vi "main_locate.vi"() -> ()   [LabVIEW 2023]
uses:
  <vilib>/Math Plots/3D Math Plots/3D Scatter/3D Scatter XCtrl/3D Scatter.xctl
  <vilib>/Math Plots/3D Math Plots/3D Scatter/3D Scatter Datatype/3D Scatter Datatype.lvclass
  subVis/datas.ctl
  subVis/HologramInfo.ctl
  HoloTrackerLib/holoTracker.lvlib
  HoloTrackerLib/CCL_parameters.ctl
  <vilib>/Math Plots/3D Math Plots/3D Scatter/3D Scatter Datatype/Public/Plot Helper (Vector).vi
  subVis/referencesBtns.ctl
  subVis/globState.vi
  <vilib>/Utility/miscctls.llb/LVStringsAndValuesArrayTypeDef_U16.ctl
  <vilib>/Python/Open Venv Python Session.vi
panel:
  out "Status":string
  in  "result tab":enum32{"Holograms", "Localisations", "infos"}(tab)
  out "2D Picture":picture caption="Hologram"
  out "3D Scatter":refnum<class "3D Plot Datatype.lvclass">[](xcontrol)
  out "Threshold":dbl
  out "Std Var":dbl
  out "Mean":dbl
  out "objects positions":sgl[][](array[numeric]) caption="objects positions\nX                           Y                         Z"
  out "t exec (ms)":u32
  in  "Tab Control":enum32{"PATH", "PARAMETERS", "ACTIONS"}(tab)=enum."ACTIONS"
  in  "HoloDir":path=path "C:/TRAVAIL/developpement/imagesHolo/1000im_manip3" caption="Holograms directory"
  in  "PythonVer":string="3.10" caption="Python version"
  in  "Python/Environnement\npath":path
  in  "remove action":enum16{"Subtract", "Division"}(ring)
  in  "Fourier BP filter (pix)":T1={"High pass (0=none)"=15.0, "Low Pass (0=none)"=125.0} {"Low Pass (0=none)" format="%#_6f"}
  in  "CCL parameters":T2={"Threshold ( N x Standard deviation)"=10.0, "Connectivity"=enum."26", "min voxel"=1.0, "max voxel"=0.0} {"max voxel" min=0.0 max=0.0; "min voxel" min=1.0 max=1.0; "Threshold ( N x Standard deviation)" min=1.0 max=100.0}
  in  "Batch threshold":T3(ring)
  in  "Focus":T4={"Type"=enum."SUM_OF_VARIANCE", "Sum size"=15} {"Sum size" min=1 max=100}
  in  "propagation":T5={"distance ini"=0.0, "number of planes"=100, "step"=1e-06} {"step" format="%#_6e"; "distance ini" format="%#_6e"}
  in  "Remove mean Hologram":bool=TRUE
  in  "HoloParam":T6 caption="Holo parameters" {"wavelength" format="%#_6e"}
  in  "hologram to test":u16(ring)
  in  "exitTestMode":bool
  in  "testMode":bool
  in  "CANCEL_BATCH":bool
  in  "EXIT":bool
  in  "BATCH":bool
  in  "Plane number":u16=95 max=200
  in  "Display":T7(ring)
  # "Analyse parameters"
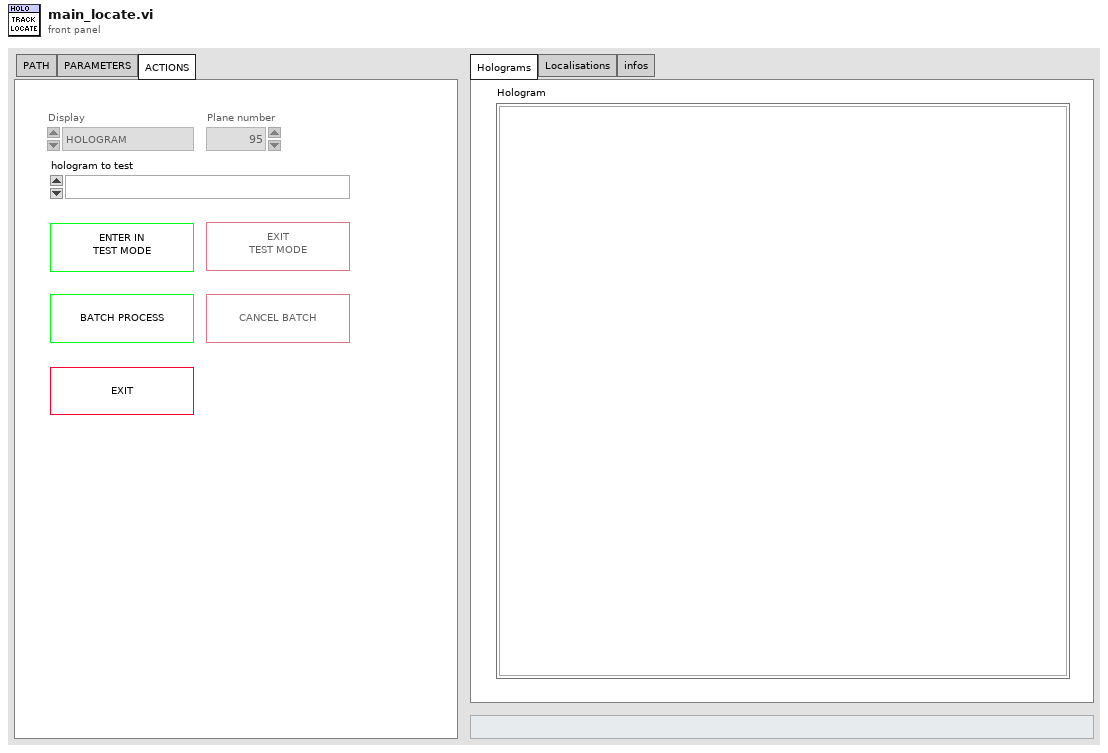
[diagram p1: front panel]
types:
  T1 = cluster{"High pass (0=none)":dbl, "Low Pass (0=none)":dbl}
  T2 = typedef "CCL_parameters.ctl" = cluster{"Threshold ( N x Standard deviation)":dbl, "Connectivity":enum16{"6", "18", "26"}, "min voxel":dbl, "max voxel":dbl}
  T3 = enum16{"compute on 1st hologram", "compute on each hologram"}
  T4 = cluster{"Type":enum16{"SUM_OF_INTENSITY", "SUM_OF_LAPLACIAN", "SUM_OF_VARIANCE", "TENENGRAD"}, "Sum size":i32}
  T5 = cluster{"distance ini":dbl, "number of planes":i32, "step":dbl}
  T6 = typedef "holoTracker.lvlib/HologramInfo.ctl" = cluster{"wavelength":sgl, "optical index":sgl, "Holo size X":i32, "Holo size Y":i32, "pixel size":sgl, "objective magnification":sgl}
  T7 = enum16{"HOLOGRAM", "XY PLANE NUMBER....", "XY MAX PLANE", "XY SUM PLANE", "XZ MAX PLANE", "XZ SUM PLANE", "YZ MAX PLANE", "YZ SUM PLANE"}
  T8 = typedef "referencesBtns.ctl" = cluster{"PythonVer":refnum<vi>, "Python/Environnement\npath":refnum<vi>, "HoloDir":refnum<vi>, "Holo parameters":refnum<vi>, "Remove mean Hologram":refnum<vi>, "propagation":refnum<vi>, "Fourier BP filter (pix)":refnum<vi>, "Focus":refnum<vi>, "Batch thresold ":refnum<vi>, "CCL parameters":refnum<vi>, "testMode":refnum<vi>, "exitTestMode":refnum<vi>, "BATCH":refnum<vi>, "CANCEL_BATCH":refnum<vi>, "EXIT":refnum<vi>, "Plane number":refnum<vi>, "Display":refnum<vi>, "remove action":refnum<vi>}
  T9 = typedef "param_defaut.ctl" = cluster{"PythonVer":string, "Python/Environnement\npath":path, "HoloDir":path, "HoloParam":T6, "Remove mean Hologram":bool, "propagation":cluster{"distance ini":dbl, "number of planes":i32, "step":dbl}, "Fourier BP filter (pix)":cluster{"High pass (0=none)":dbl, "Low Pass (0=none)":dbl}, "Focus":cluster{"Type":enum16{"SUM_OF_INTENSITY", "SUM_OF_LAPLACIAN", "SUM_OF_VARIANCE", "TENENGRAD"}, "Sum size":i32}, "Batch thresold ":enum16{"compute on 1st hologram", "compute on each hologram"}, "CCL parameters":T2}
  T10 = typedef "LVStringsAndValuesArrayTypeDef_U16.ctl" = cluster{"String":string, "Value":u16}[]
  T11 = enum16{"SESSION CLOSED", "WAIT", "TEST WAIT", "TEST IN PROGESS", "BATCH IN PROGRESS"}
  T12 = typedef "datas.ctl" = cluster{"PythonSession":refnum<k35>, "Display":bool, "BinThreshold":sgl, "LIST HOLO BATCH":path[], "Display":sgl[][], "meanHolo":sgl[][], "FEATURES(µm)":sgl[][], "LabelPicture":string, "Status":string, "planeToDisplayFeatures":enum16{"XY", "XZ", "YZ"}, "State":enum16{"SESSION CLOSED", "WAIT", "TEST WAIT", "TEST IN PROGESS", "BATCH IN PROGRESS"}, "HOLO_FILENAME":path, "HOLO_DIRECTORY":path, "LIST HOLO IN DIRECTORY":path[]}
  T13 = cluster{"Remove mean Hologram":bool, "Binarisation thresold ":enum16{"compute on 1st hologram", "compute on each hologram"}, "LIST HOLO BATCH":path[], "HoloDir":path}
  T14 = cluster{"Holo parameters":T6, "propagation":cluster{"distance ini":dbl, "number of planes":i32, "step":dbl}, "Fourier BP filter (pix)":cluster{"High pass (0=none)":dbl, "Low Pass (0=none)":dbl}, "Focus":cluster{"Type":enum16{"SUM_OF_INTENSITY", "SUM_OF_LAPLACIAN", "SUM_OF_VARIANCE", "TENENGRAD"}, "Sum size":i32}, "CCL parameters":T2}
  T15 = cluster{"Display":enum16{"HOLOGRAM", "XY PLANE NUMBER....", "XY MAX PLANE", "XY SUM PLANE", "XZ MAX PLANE", "XZ SUM PLANE", "YZ MAX PLANE", "YZ SUM PLANE"}, "Plane number":u16}
  T16 = cluster{"HOLO_array":sgl[][], "FEATURES(µm)":sgl[][], "Features(pix)":sgl[][], "planeToDisplayFeatures":enum16{"XY", "XZ", "YZ"}, "label":string}
  T17 = cluster{"X":i32, "Y":i32, "Z":i32, "XYsize":i32, "ZSize":i32}
  T18 = typedef "eventvkey.ctl" = enum16{"ASCII", "Enter", "Return", "Shift", "Ctrl", "Alt", "Cmd", "Opt", "Caps", "NumLock", "Clear", "Break", "Up", "Down", "Left", "Right", "Insert", "Delete", "Home", "End", "PageUp", "PageDown", "Escape", "Help", "Pause", "ScrollLock", "F1", "F2", "F3", "F4", "F5", "F6", "F7", "F8", "F9", "F10", "F11", "F12", "F13", "F14", "F15", "F16", "F17", "F18", "F19", "F20", "F21", "F22", "F23", "F24", "Play", "VolumeUp", "VolumeDown", "Mute", "Two Byte Char"}
  T19 = cluster{"Display":enum16{"HOLOGRAM", "XY PLANE NUMBER....", "XY MAX PLANE", "XY SUM PLANE", "XZ MAX PLANE", "XZ SUM PLANE", "YZ MAX PLANE", "YZ SUM PLANE"}, u16}
  T20 = cluster{"PythonVer":string, "Python/Environnement\npath":path, "HoloDir":path, "HoloParam":T6, "Remove mean Hologram":bool, "propagation":cluster{"distance ini":dbl, "number of planes":i32, "step":dbl}, "Fourier BP filter (pix)":cluster{"High pass (0=none)":dbl, "Low Pass (0=none)":dbl}, "Focus":cluster{"Type":enum16{"SUM_OF_INTENSITY", "SUM_OF_LAPLACIAN", "SUM_OF_VARIANCE", "TENENGRAD"}, "Sum size":i32}, "Batch threshold ":enum16{"compute on 1st hologram", "compute on each hologram"}, "CCL parameters":T2}
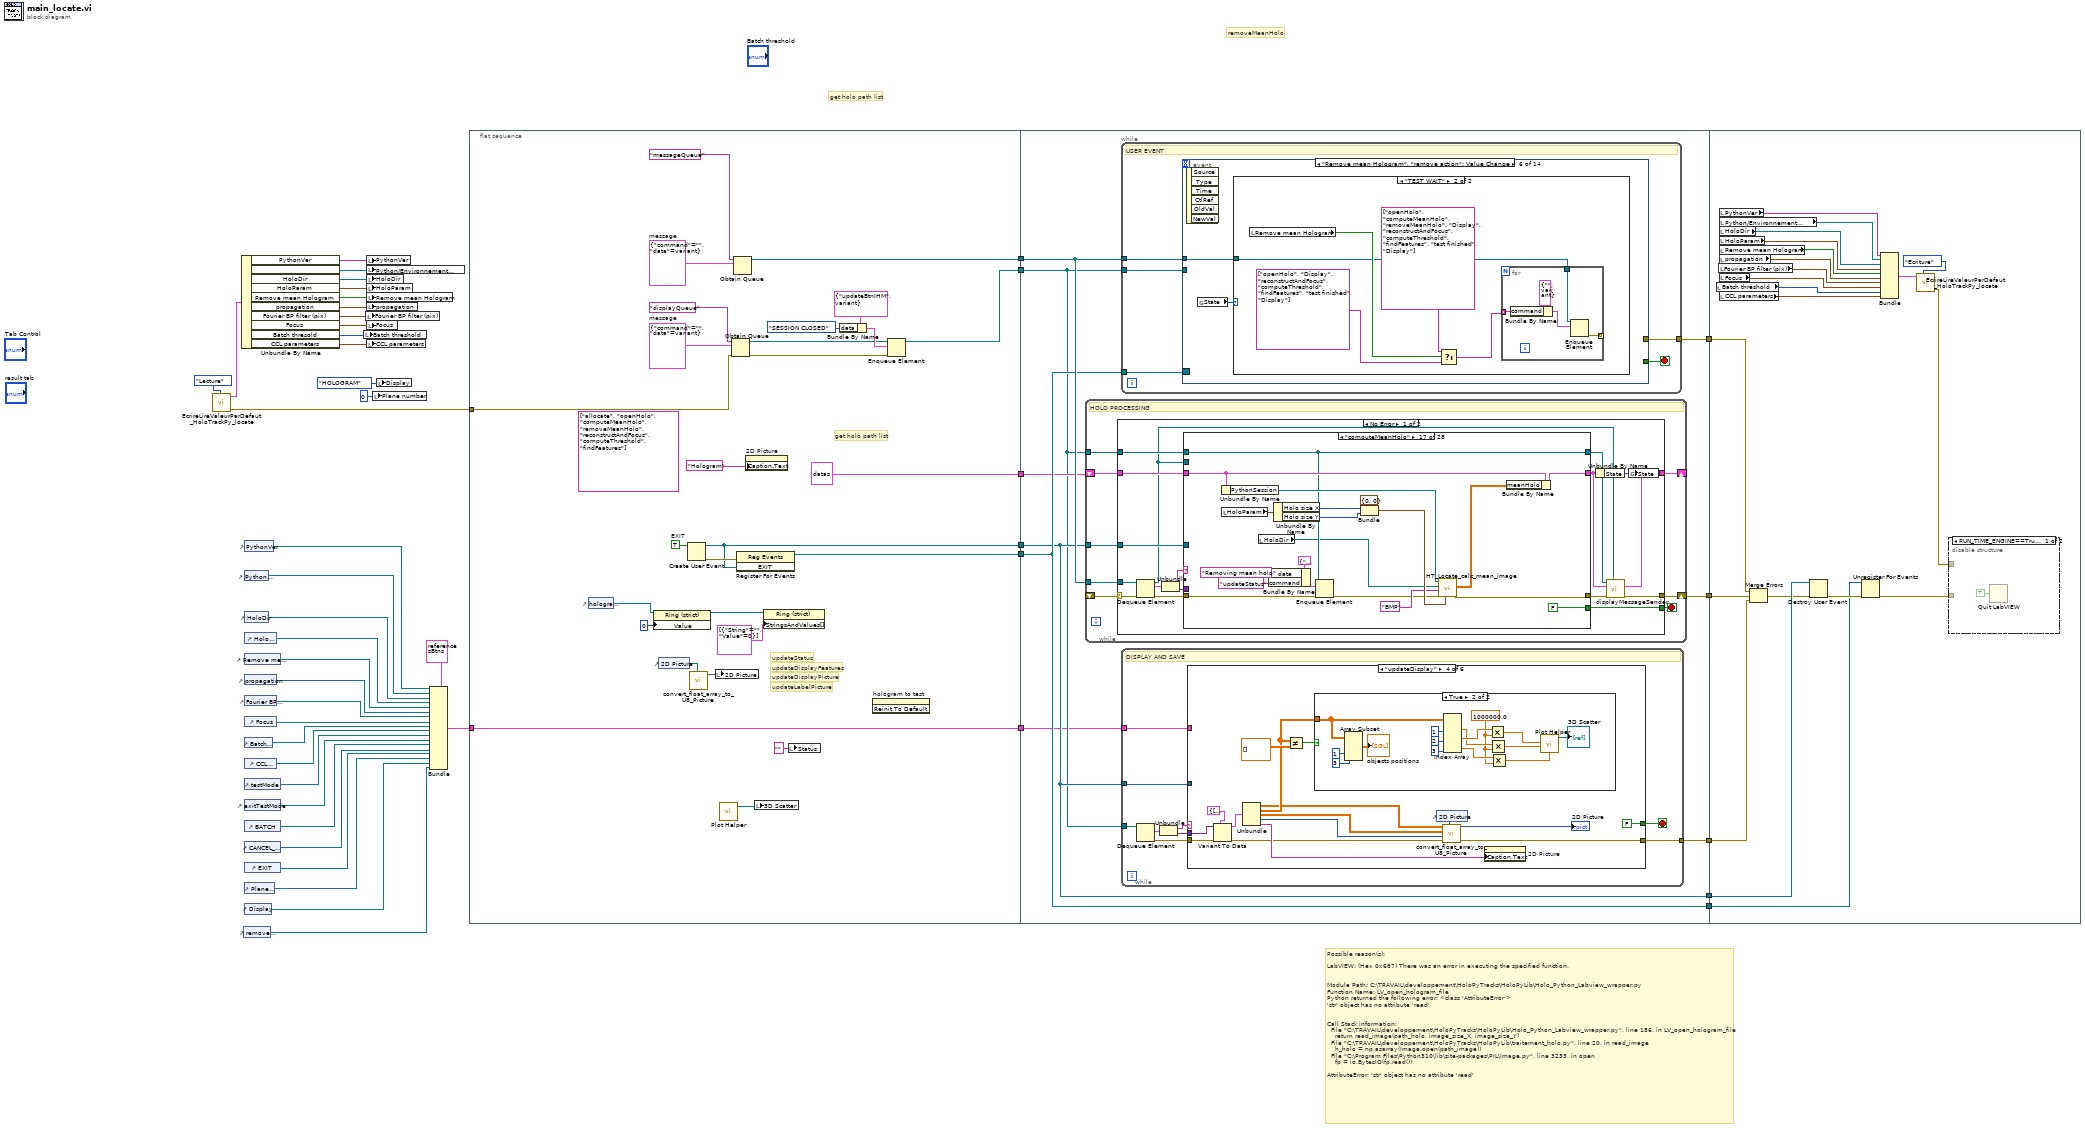
[diagram p0: block diagram]
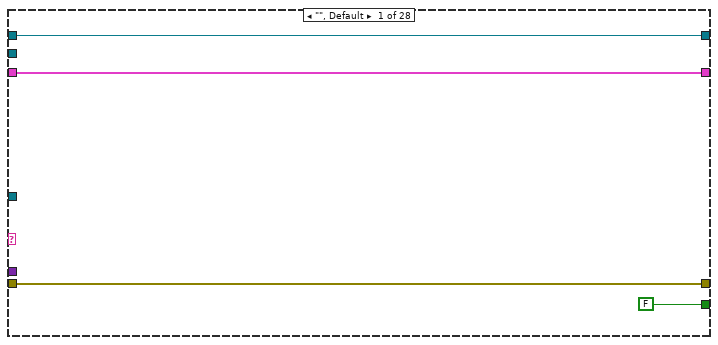
[diagram p2: hidden frame]
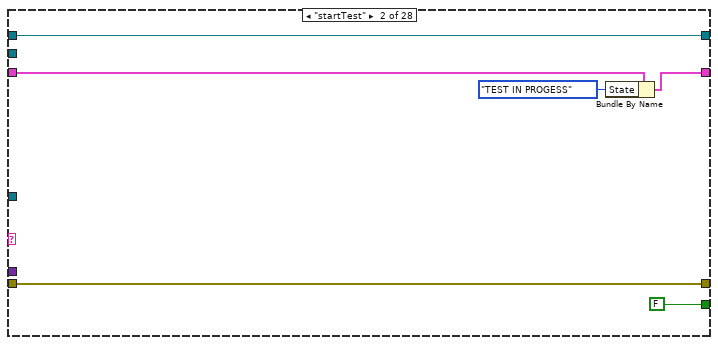
[diagram p3: hidden frame]
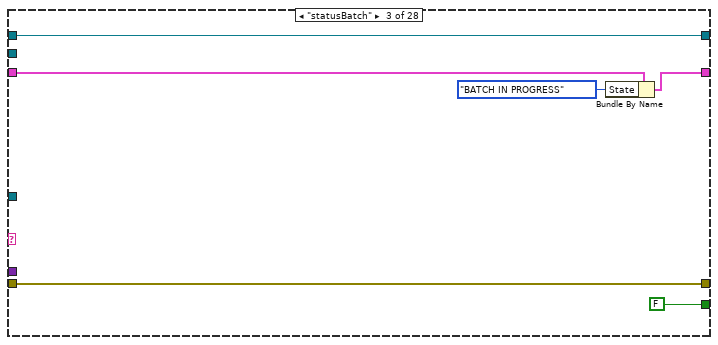
[diagram p4: hidden frame]
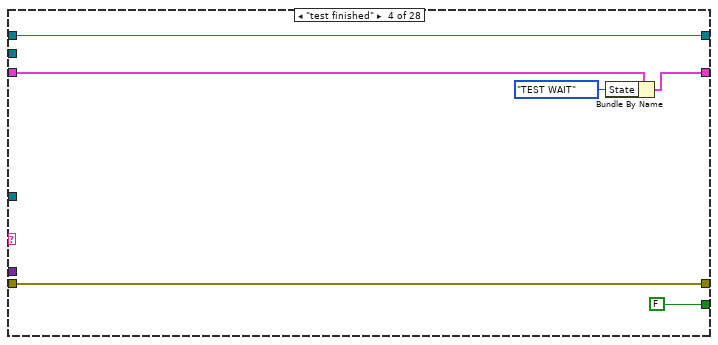
[diagram p5: hidden frame]
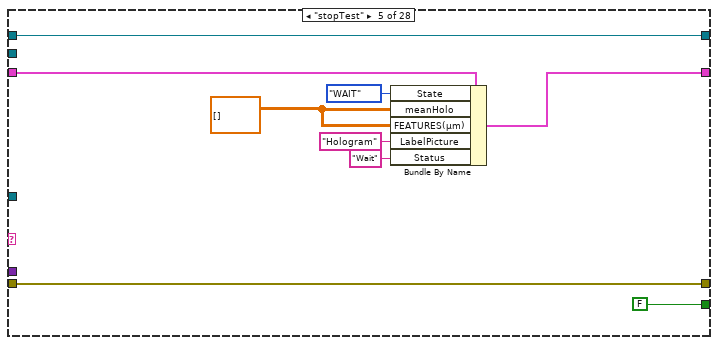
[diagram p6: hidden frame]
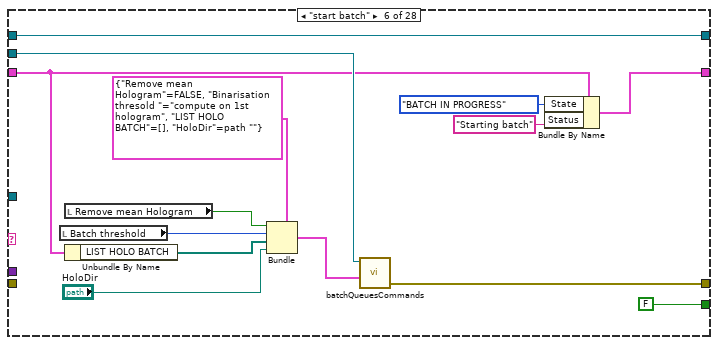
[diagram p7: hidden frame]
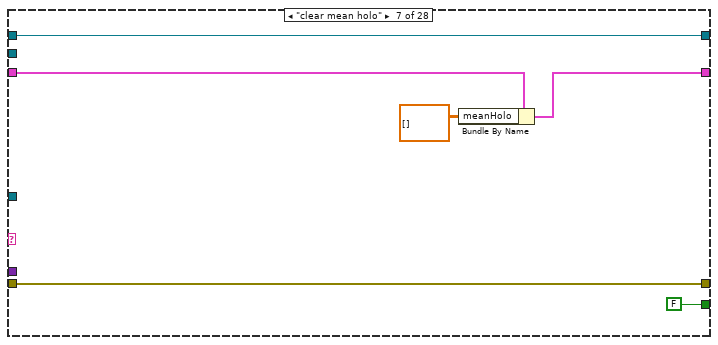
[diagram p8: hidden frame]
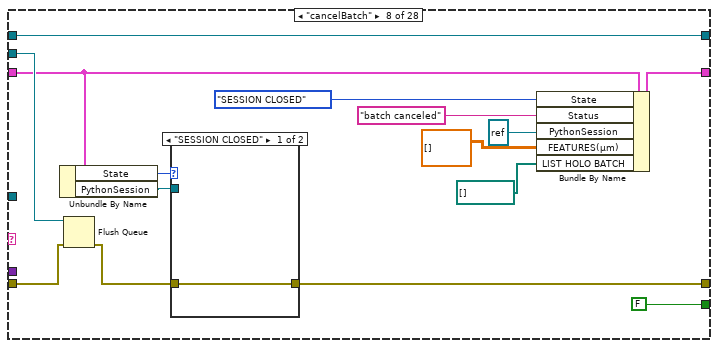
[diagram p9: hidden frame]
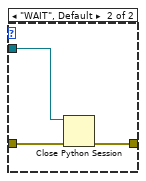
[diagram p10: hidden frame]
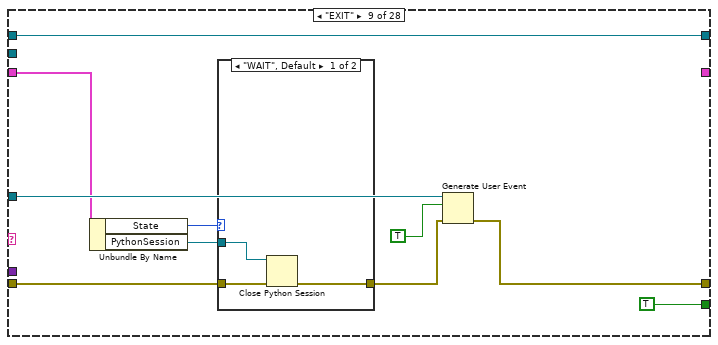
[diagram p11: hidden frame]
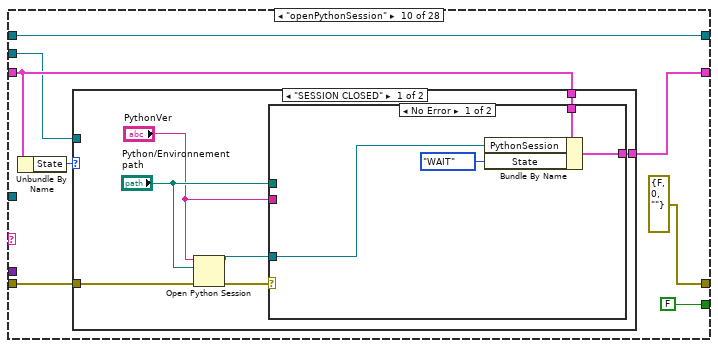
[diagram p13: hidden frame]
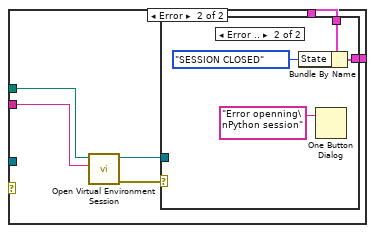
[diagram p14: hidden frame]
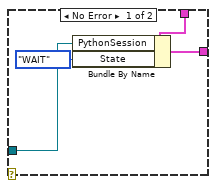
[diagram p15: hidden frame]
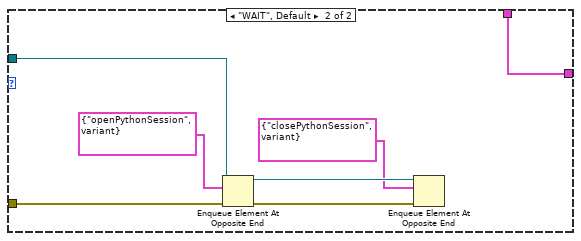
[diagram p16: hidden frame]
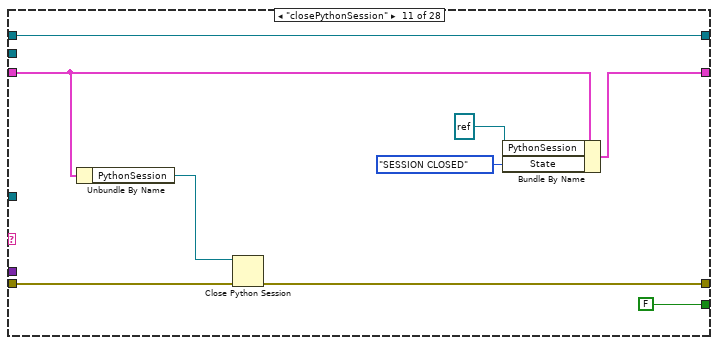
[diagram p17: hidden frame]
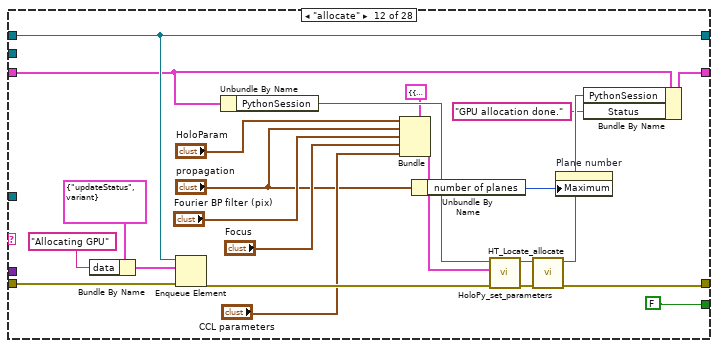
[diagram p18: hidden frame]
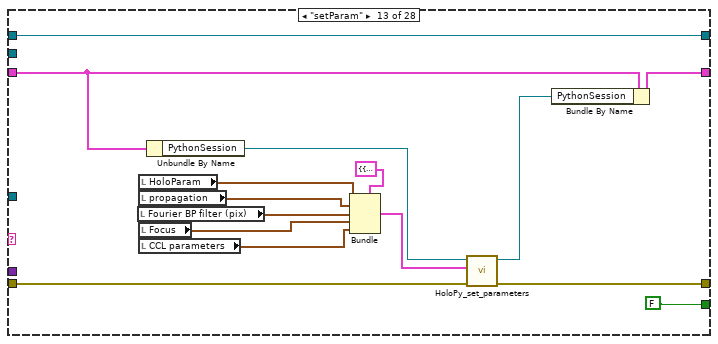
[diagram p19: hidden frame]
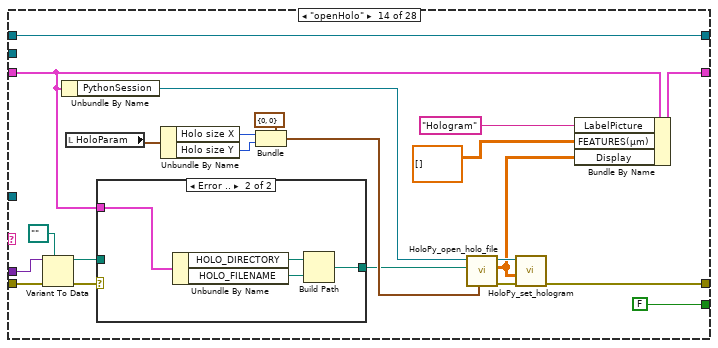
[diagram p20: hidden frame]
diagram:
  # "removeMeanHolo"
  # "get holo path list"
  # "Possible reason(s):\n\nLabVIEW: (Hex 0x687) There was an error in executing the specified function.\n\n\nModule Path: C:\\TRAVAIL\\developpement\\HoloPyTracks\\HoloPyLib\\Holo_Python_Labview_wrapper.py\nFunction Name: LV_open_hologram_file\nPython returned the following error: <class 'AttributeError'>\n'str' object has no attribute 'read'\n\n\nCall Stack information:\n  File \"C:\\TRAVAIL\\developpement\\HoloPyTracks\\HoloPyLib\\Holo_Python_Labview_wrapper.py\", line 186, in LV_open_hologram_file\n    return read_image(path_holo, image_size_X, image_size_Y)\n  File \"C:\\TRAVAIL\\developpement\\HoloPyTracks\\HoloPyLib\\traitement_holo.py\", line 20, in read_image\n    h_holo = np.asarray(Image.open(path_image))\n  File \"C:\\Program Files\\Python310\\lib\\site-packages\\PIL\\Image.py\", line 3233, in open\n    fp = io.BytesIO(fp.read())\n\nAttributeError: 'str' object has no attribute 'read'"
  n1 = call "EcrireLireValeurParDefaut_HoloTrackPy_locate.vi"("Lecture/Ecriture"=enum32{"Lecture", "Ecriture"}."Lecture") -> ("error out"=w34:errorcluster, "ParamOUT"=w36:T9)  [unwired: 7 in, 2 out]
  n2 = Unbundle By Name(w36) -> ("PythonVer"=w31:string, "Python/Environnement\npath"=w30:path, "HoloDir"=w29:path, "HoloParam"=w28:T6, "Remove mean Hologram"=w27:bool, "propagation"=w26:T5, "Fourier BP filter (pix)"=w25:T1, "Focus"=w24:T4, "Batch thresold"=w23:T3, "CCL parameters"=w22:T2)
  n3 = control-ref of="remove action"() -> (w1:refnum<vi>)
  n4 = control-ref of="Plane number"() -> (w3:refnum<vi>)
  n5 = control-ref of="Display"() -> (w2:refnum<vi>)
  n6 = control-ref of="PythonVer"() -> (w32:refnum<vi>)
  n7 = control-ref of="Python/Environnement\npath"() -> (w33:refnum<vi>)
  n8 = control-ref of="HoloDir"() -> (w16:refnum<vi>)
  n9 = control-ref of="Holo parameters"() -> (w15:refnum<vi>)
  n10 = control-ref of="Remove mean Hologram"() -> (w14:refnum<vi>)
  n11 = control-ref of="propagation"() -> (w13:refnum<vi>)
  n12 = control-ref of="Fourier BP filter (pix)"() -> (w12:refnum<vi>)
  n13 = control-ref of="Focus"() -> (w11:refnum<vi>)
  n14 = control-ref of="Batch threshold"() -> (w10:refnum<vi>)
  n15 = control-ref of="CCL parameters"() -> (w9:refnum<vi>)
  n16 = control-ref of="testMode"() -> (w8:refnum<vi>)
  n17 = control-ref of="exitTestMode"() -> (w7:refnum<vi>)
  n18 = control-ref of="BATCH"() -> (w6:refnum<vi>)
  n19 = control-ref of="CANCEL_BATCH"() -> (w5:refnum<vi>)
  n20 = control-ref of="EXIT"() -> (w4:refnum<vi>)
  n21 = local write "Batch threshold"(w23) -> ()
  n22 = local write "Fourier BP filter (pix)"(w25) -> ()
  n23 = local write "PythonVer"(w31) -> ()
  n24 = local write "Python/Environnement\npath"(w30) -> ()
  n25 = local write "HoloDir"(w29) -> ()
  n26 = local write "HoloParam"(w28) -> ()
  n27 = local write "Remove mean Hologram"(w27) -> ()
  n28 = local write "propagation"(w26) -> ()
  n29 = local write "Focus"(w24) -> ()
  n30 = local write "CCL parameters"(w22) -> ()
  n31 = local write "Plane number"(u16 0 ("Plane number")) -> ()
  n32 = local write "Display"(T7."HOLOGRAM" ("Display")) -> ()
  n33 = Bundle(cluster=T8 {"PythonVer"=refnum, "Python/Environnement\npath"=refnum, "HoloDir"=refnum, "Holo parameters"=refnum, "Remove mean Hologram"=refnum, "propagation"=refnum, "Fourier BP filter (pix)"=refnum, "Focus"=refnum, "Batch thresold "=refnum, "CCL parameters"=refnum, "testMode"=refnum, "exitTestMode"=refnum, "BATCH"=refnum, "CANCEL_BATCH"=refnum, "EXIT"=refnum, "Plane number"=refnum, "Display"=refnum, "remove action"=refnum} ("output cluster"), "PythonVer"=w32, "Python/Environnement\npath"=w33, "HoloDir"=w16, "Holo parameters"=w15, "Remove mean Hologram"=w14, "propagation"=w13, "Fourier BP filter (pix)"=w12, "Focus"=w11, "Batch thresold"=w10, "CCL parameters"=w9, "testMode"=w8, "exitTestMode"=w7, "BATCH"=w6, "CANCEL_BATCH"=w5, "EXIT"=w4, "Plane number"=w3, "Display"=w2, "remove action"=w1) -> (w20:T8)
  n34 = flat-sequence {
    tunnel: [w69] -> w46
    tunnel: [w68] -> w45
    tunnel: [w52] -> w44
    tunnel: [T12 {"PythonSession"=refnum, "Display"=FALSE, "BinThreshold"=0.0, "LIST HOLO BATCH"=[], "Display"=[], "meanHolo"=[], "FEATURES(µm)"=[], "LabelPicture"="", "Status"="", "planeToDisplayFeatures"=enum."XY", "State"=enum."SESSION CLOSED", "HOLO_FILENAME"=path "C:/TRAVAIL/developpement/imagesHolo/20um_bon_40X/20um_40x_int_.7ajp1c6t.000000.bmp", "HOLO_DIRECTORY"=path "C:/TRAVAIL/developpement/imagesHolo/20um_bon_40X/20um_40x_int_.7ajp1c6t.000000.bmp", "LIST HOLO IN DIRECTORY"=[]}] -> w43
    tunnel: [w59] -> w37
    tunnel: w20 -> [w59]
    tunnel: w34 -> [w58]
    tunnel: [w51] -> w17
    tunnel: w46 -> [w79]
    tunnel: w45 -> [w81]
    tunnel: w44 -> [w77]
    tunnel: w43 -> [w78]
    tunnel: [w81] -> w42
    tunnel: [w79] -> w41
    tunnel: [w80] -> w40
    tunnel: [w76] -> w39
    tunnel: [w75] -> w38
    tunnel: w37 -> [w74]
    tunnel: w17 -> [w82]
    tunnel: w42 -> [w964]
    tunnel: w41 -> [w963]
    tunnel: w40 -> [w960]
    tunnel: w39 -> [w962]
    tunnel: w38 -> [w961]
    frame #0 {
      (unwired) string[] ["allocate", "openHolo", "computeMeanHolo", "removeMeanHolo", "reconstructAndFocus", "computeThreshold", "findFeatures"]
      w67 = cluster{"command":string, "data":variant} {"command"="", "data"=variant}  # message
      w71 = TRUE  # EXIT
      w72 = cluster{"command":string, "data":variant} {"command"="", "data"=variant}  # message
      # "get holo path list"
      # "updateDisplayFeatures"
      # "updateLabelPicture"
      # "updateDisplayPicture"
      # "updateStatus"
      n35 = control-ref of="hologram to test"() -> (w48:refnum<vi>)
      n36 = property class="Ring (strict)"(reference=w48, "Value"=u16 0) -> (reference out=w47:refnum<vi>)  [unwired: 1 in, 1 out]
      n37 = control-ref of="2D Picture"() -> (w64:refnum<vi>)
      n38 = Create User Event(user event datatype=w71) -> (user event=w69:refnum<user-event>, error out=w70:errorcluster)  [unwired: 1 in]
      n39 = call "convert_float_array_to_U8_Picture.vi"("Pict Refnum"=w64) -> ("new picture"=w63:picture)  [unwired: 9 in, 1 out]
      n40 = local write "2D Picture"(w63) -> ()
      n41 = call-poly <vilib>:"Plot Helper.vi"() -> ("3D Plot lvclass Array out"=w60:refnum<class "3D Plot Datatype.lvclass">[])  [unwired: 6 in, 5 out]
      n42 = Obtain Queue(name (unnamed)="displayQueue", element data type=w67, error in (no error)=w58) -> (queue out=w55:refnum<queue>, error out=w54:errorcluster)  [unwired: 2 in, 1 out]
      n43 = Obtain Queue(name (unnamed)="messageQueue", element data type=w72) -> (queue out=w51:refnum<queue>)  [unwired: 3 in, 2 out]
      n44 = register-events(error in=w70, w69) -> (reference out=w68:refnum<event-registration>)  [unwired: 1 in, 1 out]
      n45 = property on="2D Picture" class="Pict"("Caption.Text"="Hologram" ("Label.Text")) -> ()  [unwired: 2 in, 2 out]
      n46 = local write "3D Scatter"(w60) -> ()
      n47 = property class="Ring (strict)"(reference=w47, "StringsAndValues[]"=T10 [{"String"="", "Value"=0}] ("Strings And Values []")) -> ()  [unwired: 1 in, 2 out]
      n48 = local write "Status"("" ("Status")) -> ()
      n49 = Bundle By Name(cluster=cluster{"command":string, "data":variant} {"command"="updateBtnIHM", "data"=variant} ("element"), "data"=T11."SESSION CLOSED" ("State")) -> (w56:cluster{"command":string, "data":variant})
      n50 = invoke on="hologram to test" class="Ring (strict)" method="Reinit To Default"() -> ()  [unwired: 3 in, 3 out]
      n51 = Enqueue Element(queue=w55, element=w56, error in (no error)=w54) -> (queue out=w52:refnum<queue>)  [unwired: 1 in, 2 out]
    }
    frame #1 {
      n52 = while {
        tunnel: w82 -> [w90]
        tunnel: w79 -> [w88]
        shift-right: [w86] -> _
        shift-left: w78 -> [w87]
        tunnel: w77 -> [w85]
        shift-right: [w84] -> w75
        shift-left: _ -> [w83]
        stop <- w89 stop-if-true
        # "HOLO PROCESSING"
        n53 = case shown="No Error" w83 {
          selector: w83 -> [w98 w699]
          tunnel: w90 -> [w107 w700]
          tunnel: [w102 FALSE] -> w89
          tunnel: w88 -> [w101 _]
          tunnel: w87 -> [w100 w695]
          tunnel: [w94 w695] -> w86
          tunnel: w85 -> [w99 _]
          tunnel: [w96 errorcluster {"status"=FALSE, "code"=0, "source"=""} ("error out")] -> w84
          frame No Error {
            n54 = Dequeue Element(queue=w107, error in (no error)=w98) -> (queue out=w91:refnum<queue>, element=w105:cluster{"command":string, "data":variant}, error out=w106:errorcluster)  [unwired: 1 in, 1 out]
            n55 = Unbundle(w105) -> ("command"=w104:string, "data"=w103:variant)
            n56 = case shown="\"computeMeanHolo\"" w104 {
              tunnel: w106 -> [w109 w113 w119 w125 w131 _ w154 w169 w183 w197 w236 w259 w273 w285 w313 w320 w336 w352 w378 w389 w411 w448 w621 w633 w656 w672 w676 w693]
              tunnel: w103 -> [_ _ _ _ _ _ _ _ _ _ _ _ _ w284 _ _ _ _ _ _ w410 w447 _ w632 w655 w671 _ w692]
              tunnel: [FALSE FALSE FALSE FALSE FALSE FALSE FALSE FALSE TRUE FALSE FALSE FALSE FALSE FALSE FALSE FALSE FALSE FALSE FALSE FALSE FALSE FALSE FALSE FALSE FALSE FALSE FALSE FALSE] -> w102
              tunnel: w101 -> [_ _ _ _ _ _ _ _ w186 _ _ _ _ _ _ _ _ _ _ _ _ _ _ _ _ _ _ _]
              tunnel: w100 -> [w110 w115 w121 w127 w136 w146 w157 w163 w178 w193 w235 w256 w272 w279 w317 w324 w342 w358 w375 w387 w406 w451 w625 w639 w651 w670 w682 w686]
              tunnel: [w110 w114 w120 w126 w135 w148 w156 w172 _ w196 w237 w262 w277 w296 w318 w326 w341 w357 w374 w386 w405 w451 w624 w638 w650 w669 w681 w686] -> w93
              tunnel: w99 -> [w108 w116 w122 w128 w137 w149 w158 w168 w179 w198 w239 w258 w276 w293 w314 w325 w334 w356 w376 w385 w407 w450 w626 w640 w649 w668 w680 w684]
              tunnel: [w109 w113 w119 w125 w131 w150 w154 w161 w180 errorcluster {"status"=FALSE, "code"=0, "source"=""} ("error out") w233 w254 w275 w291 w310 w320 w335 w355 w373 w388 w394 w452 w620 w635 w644 w660 w679 w689] -> w95
              tunnel: w91 -> [_ _ _ _ _ w151 _ w170 _ w192 _ _ _ _ _ _ _ _ _ _ _ _ _ _ _ _ _ _]
              tunnel: [w108 w116 w122 w128 w137 w149 w158 w168 w179 w198 w239 w258 w276 w293 w314 w325 w334 w356 w376 w385 w407 w450 w626 w640 w649 w668 w680 w684] -> w97
              frame "", Default {
              }
              frame "startTest" {
                n57 = Bundle By Name(cluster=w115, "State"=T11."TEST IN PROGESS") -> (w114:T12)
              }
              frame "statusBatch" {
                n58 = Bundle By Name(cluster=w121, "State"=T11."BATCH IN PROGRESS") -> (w120:T12)
              }
              frame "test finished" {
                n59 = Bundle By Name(cluster=w127, "State"=T11."TEST WAIT") -> (w126:T12)
              }
              frame "stopTest" {
                w132 = sgl[][] [] ("meanHolo")
                n60 = Bundle By Name(cluster=w136, "State"=T11."WAIT", "meanHolo"=w132, "FEATURES(µm)"=w132, "LabelPicture"="Hologram", "Status"="Wait") -> (w135:T12)
              }
              frame "start batch" {
                n61 = local read "Batch threshold"() -> (w144:T3)
                n62 = local read "Remove mean Hologram"() -> (w145:bool)
                n63 = Unbundle By Name(w146) -> ("LIST HOLO BATCH"=w143:path[])
                n64 = Bundle(cluster=T13 {"Remove mean Hologram"=FALSE, "Binarisation thresold "=enum."compute on 1st hologram", "LIST HOLO BATCH"=[], "HoloDir"=path ""} ("Batch parameters"), "Remove mean Hologram"=w145, "Binarisation thresold"=w144, "LIST HOLO BATCH"=w143, "HoloDir"="HoloDir") -> (w142:T13)
                n65 = call "batchQueuesCommands.vi"("Batch parameters"=w142, "QueueMessages"=w151) -> ("error out"=w150:errorcluster)  [unwired: 9 in]
                n66 = Bundle By Name(cluster=w146, "State"=T11."BATCH IN PROGRESS", "Status"="Starting batch") -> (w148:T12)
              }
              frame "clear mean holo" {
                n67 = Bundle By Name(cluster=w157, "meanHolo"=sgl[][] []) -> (w156:T12)
              }
              frame "cancelBatch" {
                n68 = Unbundle By Name(w163) -> ("State"=w162:T11, "PythonSession"=w159:refnum<k35>)
                n69 = Flush Queue(queue=w170, error in (no error)=w169) -> (error out=w160:errorcluster)  [unwired: 2 out]
                n70 = case shown="\"SESSION CLOSED\"" w162 {
                  tunnel: [w174 w175] -> w161
                  tunnel: w160 -> [w174 w177]
                  tunnel: w159 -> [_ w176]
                  frame "SESSION CLOSED" {
                  }
                  frame "WAIT", Default {
                    n71 = Close Python Session(session in=w176, error in=w177) -> (11:w175:errorcluster)
                  }
                }
                n72 = Bundle By Name(cluster=w163, "State"=T11."SESSION CLOSED", "Status"="batch canceled" ("command"), "PythonSession"=refnum<k35> refnum, "FEATURES(µm)"=sgl[][] [] ("Holo"), "LIST HOLO BATCH"=path[] []) -> (w172:T12)
              }
              frame "EXIT" {
                n73 = Unbundle By Name(w178) -> ("State"=w184:T11, "PythonSession"=w182:refnum<k35>)
                n74 = case shown="\"WAIT\", Default" w184 {
                  tunnel: w183 -> [w190 w191]
                  tunnel: w182 -> [w189 _]
                  tunnel: [w188 w191] -> w181
                  frame "WAIT", Default {
                    n75 = Close Python Session(session in=w189, error in=w190) -> (11:w188:errorcluster)
                  }
                  frame "SESSION CLOSED" {
                  }
                }
                n76 = Generate User Event(user event=w186, event data cluster=TRUE ("event data"), error in=w181) -> (error out=w180:errorcluster)  [unwired: 1 in, 1 out]
              }
              frame "openPythonSession" {
                n77 = Unbundle By Name(w193) -> ("State"=w194:T11)
                n78 = case shown="\"SESSION CLOSED\"" w194 {
                  tunnel: w197 -> [w206 w231]
                  tunnel: [w203 w225] -> w196
                  tunnel: w193 -> [w200 w225]
                  tunnel: w192 -> [_ w230]
                  frame "SESSION CLOSED" {
                    n79 = Open Python Session(python version="PythonVer", python path="Python/Environnement\npath", 3:w206) -> (session out=w202:refnum<k35>, error out=w205:errorcluster)
                    n80 = case shown="No Error" w205 {
                      tunnel: "Python/Environnement\npath" -> [_ w216]
                      tunnel: "PythonVer" -> [_ w215]
                      tunnel: w200 -> [w210 w213]
                      tunnel: [w209 w212] -> w203
                      tunnel: w202 -> [w208 _]
                      frame No Error {
                        n81 = Bundle By Name(cluster=w210, "PythonSession"=w208, "State"=T11."WAIT") -> (w209:T12)
                      }
                      frame Error {
                        n82 = call-poly <vilib>:"Open Virtual Environment Session.vi"("Python version"=w215, "Env path"=w216) -> ("error out"=w214:errorcluster, "session out"=w211:refnum<k35>)  [unwired: 8 in]
                        n83 = case shown="Error .." w214 {
                          tunnel: w213 -> [w220 w223]
                          tunnel: [w219 w222] -> w212
                          tunnel: w211 -> [w218 _]
                          frame No Error {
                            n84 = Bundle By Name(cluster=w220, "PythonSession"=w218, "State"=T11."WAIT") -> (w219:T12)
                          }
                          frame Error {
                            n85 = Bundle By Name(cluster=w223, "State"=T11."SESSION CLOSED") -> (w222:T12)
                            n86 = One Button Dialog(message="Error openning\nPython session") -> ()  [unwired: 1 in, 1 out]
                          }
                        }
                      }
                    }
                  }
                  frame "WAIT", Default {
                    n87 = Enqueue Element At Opposite End(queue=w230, element=cluster{"command":string, "data":variant} {"command"="openPythonSession", "data"=variant}, error in (no error)=w231) -> (queue out=w227:refnum<queue>, error out=w228:errorcluster)  [unwired: 1 in, 1 out]
                    n88 = Enqueue Element At Opposite End(queue=w227, element=cluster{"command":string, "data":variant} {"command"="closePythonSession", "data"=variant}, error in (no error)=w228) -> ()  [unwired: 1 in, 3 out]
                  }
                }
              }
              frame "closePythonSession" {
                n89 = Unbundle By Name(w235) -> ("PythonSession"=w234:refnum<k35>)
                n90 = Close Python Session(session in=w234, error in=w236) -> (11:w233:errorcluster)
                n91 = Bundle By Name(cluster=w235, "PythonSession"=refnum<k35> refnum, "State"=T11."SESSION CLOSED") -> (w237:T12)
              }
              frame "allocate" {
                n92 = Bundle By Name(cluster=cluster{"command":string, "data":variant} {"command"="updateStatus", "data"=variant} ("element"), "data"="Allocating GPU" ("command")) -> (w257:cluster{"command":string, "data":variant})
                n93 = Enqueue Element(queue=w258, element=w257, error in (no error)=w259) -> (error out=w252:errorcluster)  [unwired: 1 in, 2 out]
                n94 = Unbundle By Name(w256) -> ("PythonSession"=w250:refnum<k35>)
                n95 = Bundle(cluster=T14 {"Holo parameters"={"wavelength"=0.0, "optical index"=0.0, "Holo size X"=0, "Holo size Y"=0, "pixel size"=0.0, "objective magnification"=0.0}, "propagation"={"distance ini"=0.0, "number of planes"=0, "step"=0.0}, "Fourier BP filter (pix)"={"High pass (0=none)"=0.0, "Low Pass (0=none)"=0.0}, "Focus"={"Type"=enum."SUM_OF_INTENSITY", "Sum size"=0}, "CCL parameters"={"Threshold ( N x Standard deviation)"=0.0, "Connectivity"=enum."6", "min voxel"=0.0, "max voxel"=0.0}} ("ParametersIN"), "Holo parameters"="HoloParam", "propagation"="propagation", "Fourier BP filter (pix)"="Fourier BP filter (pix)", "Focus"="Focus", "CCL parameters"="CCL parameters") -> (w248:T14)
                n96 = Unbundle By Name("propagation") -> ("number of planes"=w241:i32)
                n97 = call "HoloPy_set_parameters.vi"("error in (no error)"=w252, "ParametersIN"=w248, "session in"=w250) -> ("error out"=w251:errorcluster, "Refnum out"=w249:refnum<k35>)  [unwired: 6 in, 1 out]
                n98 = call "HT_Locate_allocate.vi"("error in (no error)"=w251, "session in"=w249) -> ("error out"=w254:errorcluster, "Refnum out"=w255:refnum<k35>)  [unwired: 7 in, 1 out]
                n99 = property on="Plane number" class="DigNum (strict)"("Maximum"=w241) -> ()  [unwired: 2 in, 2 out]
                n100 = Bundle By Name(cluster=w256, "PythonSession"=w255, "Status"="GPU allocation done." ("command")) -> (w262:T12)
              }
              frame "setParam" {
                n101 = local read "Fourier BP filter (pix)"() -> (w267:T1)
                n102 = local read "HoloParam"() -> (w269:T6)
                n103 = local read "propagation"() -> (w268:T5)
                n104 = local read "Focus"() -> (w266:T4)
                n105 = local read "CCL parameters"() -> (w265:T2)
                n106 = Unbundle By Name(w272) -> ("PythonSession"=w271:refnum<k35>)
                n107 = Bundle(cluster=T14 {"Holo parameters"={"wavelength"=0.0, "optical index"=0.0, "Holo size X"=0, "Holo size Y"=0, "pixel size"=0.0, "objective magnification"=0.0}, "propagation"={"distance ini"=0.0, "number of planes"=0, "step"=0.0}, "Fourier BP filter (pix)"={"High pass (0=none)"=0.0, "Low Pass (0=none)"=0.0}, "Focus"={"Type"=enum."SUM_OF_INTENSITY", "Sum size"=0}, "CCL parameters"={"Threshold ( N x Standard deviation)"=0.0, "Connectivity"=enum."6", "min voxel"=0.0, "max voxel"=0.0}} ("ParametersIN"), "Holo parameters"=w269, "propagation"=w268, "Fourier BP filter (pix)"=w267, "Focus"=w266, "CCL parameters"=w265) -> (w270:T14)
                n108 = call "HoloPy_set_parameters.vi"("error in (no error)"=w273, "ParametersIN"=w270, "session in"=w271) -> ("error out"=w275:errorcluster, "Refnum out"=w274:refnum<k35>)  [unwired: 6 in, 1 out]
                n109 = Bundle By Name(cluster=w272, "PythonSession"=w274) -> (w277:T12)
              }
              frame "openHolo" {
                n110 = Variant To Data(error in=w285, type=path "" ("appended path"), Variant=w284) -> (data=w280:path, error out=w282:errorcluster)
                n111 = Unbundle By Name(w279) -> ("PythonSession"=w299:refnum<k35>)
                n112 = local read "HoloParam"() -> (w289:T6)
                n113 = case shown="Error .." w282 {
                  tunnel: [w301 w302] -> w281
                  tunnel: w280 -> [w301 _]
                  tunnel: w279 -> [_ w305]
                  frame No Error {
                  }
                  frame Error {
                    n114 = Unbundle By Name(w305) -> ("HOLO_DIRECTORY"=w304:path, "HOLO_FILENAME"=w303:path)
                    n115 = Build Path(base path=w304, name or relative path=w303) -> (appended path=w302:path)
                  }
                }
                n116 = Unbundle By Name(w289) -> ("Holo size X"=w288:i32, "Holo size Y"=w287:i32)
                n117 = Bundle(cluster=cluster{"image_size_X":i32, "image_size_Y":i32} {"image_size_X"=0, "image_size_Y"=0} ("imageSize"), "image_size_X"=w288, "image_size_Y"=w287) -> (w297:cluster{"image_size_X":i32, "image_size_Y":i32})
                n118 = call "HoloPy_open_holo_file.vi"("imageSize"=w297, "image path"=w281, "Refnum in"=w299) -> ("error out"=w295:errorcluster, "Array"=w286:sgl[][], "Refnum out"=w294:refnum<k35>)  [unwired: 6 in]
                n119 = call "HoloPy_set_hologram.vi"("error in (no error)"=w295, "HOLO_array"=w286, "Refnum in"=w294) -> ("error out"=w291:errorcluster)  [unwired: 6 in, 2 out]
                n120 = Bundle By Name(cluster=w279, "LabelPicture"="Hologram" ("Label.Text"), "FEATURES(µm)"=sgl[][] [], "Display"=w286) -> (w296:T12)
              }
              frame "get holo path list" {
                n121 = Unbundle By Name(w317) -> ("PythonSession"=w316:refnum<k35>)
                n122 = local read "HoloDir"() -> (w308:path)
                n123 = call "HoloPy_get_all_image_files_in_directory.vi"("error in (no error)"=w313, "file_extension"="BMP", "holo directory"=w308, "Refnum in"=w316) -> ("error out"=w311:errorcluster, "path"=w306:path[], "Refnum out"=w307:refnum<k35>)  [unwired: 5 in]
                n124 = Index Array(array=w306) -> (element=w309:path)  [unwired: 1 in]
                n125 = control-ref of="hologram to test"() -> (w312:refnum<vi>)
                n126 = call "displayHoloListEnum.vi"("error in (no error)"=w311, "path"=w306, "Ring in"=w312) -> ("error out"=w310:errorcluster)  [unwired: 8 in]
                n127 = Bundle By Name(cluster=w317, "PythonSession"=w307, "LIST HOLO IN DIRECTORY"=w306, "LIST HOLO BATCH"=w306, "HOLO_FILENAME"=w309, "HOLO_DIRECTORY"=w308) -> (w318:T12)
              }
              frame "change holo" {
                n128 = Unbundle By Name(w324) -> ("LIST HOLO IN DIRECTORY"=w323:path[])
                n129 = Index Array(array=w323, index="hologram to test") -> (element=w321:path)
                n130 = Bundle By Name(cluster=w324, "HOLO_FILENAME"=w321) -> (w326:T12)
              }
              frame "computeMeanHolo" {
                n131 = Unbundle By Name(w342) -> ("PythonSession"=w344:refnum<k35>)
                n132 = local read "HoloParam"() -> (w332:T6)
                n133 = local read "HoloDir"() -> (w329:path)
                n134 = Bundle By Name(cluster=cluster{"command":string, "data":variant} {"command"="", "data"=variant} ("element"), "data"="Removing mean holo" ("command"), "command"="updateStatus") -> (w338:cluster{"command":string, "data":variant})
                n135 = Unbundle By Name(w332) -> ("Holo size X"=w331:i32, "Holo size Y"=w330:i32)
                n136 = Enqueue Element(queue=w334, element=w338, error in (no error)=w336) -> (error out=w333:errorcluster)  [unwired: 1 in, 2 out]
                n137 = Bundle(cluster=cluster{"image_size_X":i32, "image_size_Y":i32} {"image_size_X"=0, "image_size_Y"=0} ("imageSize"), "image_size_X"=w331, "image_size_Y"=w330) -> (w345:cluster{"image_size_X":i32, "image_size_Y":i32})
                n138 = call "HT_Locate_calc_mean_image.vi"("imageSize"=w345, "error in (no error)"=w333, "imageFileExtension"="BMP", "directory path"=w329, "Refnum in"=w344) -> ("error out"=w335:errorcluster, "Array"=w328:sgl[][])  [unwired: 4 in, 1 out]
                n139 = Bundle By Name(cluster=w342, "meanHolo"=w328) -> (w341:T12)
              }
              frame "removeMeanHolo" {
                n140 = Unbundle By Name(w358) -> ("PythonSession"=w360:refnum<k35>, "meanHolo"=w359:sgl[][])
                n141 = call "HoloPy_get_hologram.vi"("error in (no error)"=w352, "Refnum in"=w360) -> ("error out"=w362:errorcluster, "HOLO_array"=w348:sgl[][], "Refnum out"=w361:refnum<k35>)  [unwired: 7 in]
                n142 = case shown="\"Division\"" "remove action" {
                  tunnel: w348 -> [w368 w371]
                  tunnel: w359 -> [w367 w370]
                  tunnel: [w364 w369] -> w350
                  frame "Subtract", Default {
                    n143 = Subtract(x=w368, y=w367) -> (x-y=w366:sgl[][])
                    n144 = Array Max & Min(array=w366) -> (min value=w365:sgl)  [unwired: 3 out]
                    n145 = Subtract(x=w366, y=w365) -> (x-y=w364:sgl[][])
                  }
                  frame "Division" {
                    n146 = Divide(x=w371, y=w370) -> (x/y=w369:sgl[][])
                  }
                }
                n147 = call "HoloPy_set_hologram.vi"("error in (no error)"=w362, "HOLO_array"=w350, "Refnum in"=w361) -> ("error out"=w355:errorcluster, "Refnum out"=w351:refnum<k35>)  [unwired: 6 in, 1 out]
                n148 = Bundle By Name(cluster=w358, "PythonSession"=w351, "LabelPicture"="Hologram", "planeToDisplayFeatures"=enum16{"XY", "XZ", "YZ"}."XY", "Display"=w350) -> (w357:T12)
              }
              frame "reconstructAndFocus" {
                n149 = Unbundle By Name(w375) -> ("PythonSession"=w377:refnum<k35>)
                n150 = call "HoloPy_volume_and_focus.vi"("error in (no error)"=w378, "Refnum in"=w377) -> ("error out"=w373:errorcluster, "Refnum out"=w372:refnum<k35>)  [unwired: 7 in, 1 out]
                n151 = Bundle By Name(cluster=w375, "PythonSession"=w372) -> (w374:T12)
              }
              frame "computeThreshold" {
                n152 = local read "CCL parameters"() -> (w384:T2)
                n153 = Unbundle By Name(w387) -> ("PythonSession"=w392:refnum<k35>)
                n154 = Unbundle By Name(w384) -> ("Threshold ( N x Standard deviation)"=w383:dbl)
                n155 = call "HoloPy_get_mean_std_var_volume.vi"("error in (no error)"=w389, "Refnum in"=w392) -> ("error out"=w388:errorcluster, "data volume"=w391:cluster{"mean":dbl, "std var":dbl})  [unwired: 7 in, 1 out]
                n156 = Unbundle By Name(w391) -> ("mean"=w380:dbl, "std var"=w382:dbl)
                "Std Var" <- w382
                "Mean" <- w380
                n157 = Multiply(x=w383, y=w382) -> (x*y=w390:dbl)
                n158 = Add(x=w380, y=w390) -> (x+y=w381:dbl)
                "Threshold" <- w381
                n159 = Bundle By Name(cluster=w387, "BinThreshold"=w381) -> (w386:T12)
              }
              frame "findFeatures" {
                n160 = Unbundle By Name(w406) -> ("LIST HOLO BATCH"=w403:path[], "PythonSession"=w408:refnum<k35>, "BinThreshold"=w409:sgl)
                n161 = Variant To Data(error in=w411, type=cluster{"imageNumber":u32, "Display":bool} {"imageNumber"=0, "Display"=TRUE}, Variant=w410) -> (data=w398:cluster{"imageNumber":u32, "Display":bool}, error out=w399:errorcluster)
                n162 = case shown="Error .." w399 {
                  tunnel: w398 -> [w418 _]
                  tunnel: [w417 u32 0 ("imageNumber")] -> w397
                  tunnel: [w416 TRUE ("Display")] -> w396
                  frame No Error {
                    n163 = Unbundle(w418) -> ("imageNumber"=w417:u32, "Display"=w416:bool)
                  }
                  frame Error {
                  }
                }
                n164 = Array Size(array=w403) -> (size(s)=w400:i32)
                n165 = Equal To 0?(x=w397) -> (x = 0?=w402:bool)
                n166 = call "HoloPy_Find_Features.vi"("imageNumber"=w397, "Threshold"=w409, "Refnum in"=w408) -> ("error out"=w394:errorcluster, "FEATURES(µm)"=w395:sgl[][])  [unwired: 6 in, 1 out]
                n167 = case shown="True" w402 {
                  tunnel: w395 -> [w426 w439]
                  tunnel: [w421 w427] -> w401
                  tunnel: w397 -> [_ w435]
                  tunnel: w400 -> [_ w436]
                  frame True {
                    n168 = Array Size(array=w426) -> (size(s)=w425:i32[])
                    n169 = Index Array(array=w425) -> (element=w424:i32)  [unwired: 1 in]
                    n170 = Number To Decimal String(number=w424) -> (decimal integer string=w422:string)  [unwired: 1 in]
                    n171 = Concatenate Strings(w422, " features found.") -> (w421:string)
                  }
                  frame False {
                    n172 = Array Size(array=w439) -> (size(s)=w438:i32[])
                    n173 = Number To Decimal String(number=w436) -> (decimal integer string=w431:string)  [unwired: 1 in]
                    n174 = Number To Decimal String(number=w435) -> (decimal integer string=w433:string)  [unwired: 1 in]
                    n175 = Index Array(array=w438) -> (element=w437:i32)  [unwired: 1 in]
                    n176 = Number To Decimal String(number=w437) -> (decimal integer string=w429:string)  [unwired: 1 in]
                    n177 = Concatenate Strings("Holo n°", w433, "/", w431, ". " ("string"), w429, " features found.") -> (w427:string)
                  }
                }
                n178 = flat-sequence {
                  tunnel: w394 -> [_]
                  frame #0 {
                    n179 = Tick Count (ms)() -> (millisecond timer value=w414:u32)
                    n180 = feedback #1() -> (w415:u32)  [unwired: 1 in]
                    n181 = feedback-in #1(w414) -> ()
                    n182 = Subtract(x=w414, y=w415) -> (x-y=→"t exec (ms)":u32)
                  }
                }
                n183 = Bundle By Name(cluster=w406, "FEATURES(µm)"=w395, "Display"=w396, "Status"=w401) -> (w405:T12)
              }
              frame "Display" {
                n184 = Unbundle By Name(w451) -> ("PythonSession"=w453:refnum<k35>, "FEATURES(µm)"=w449:sgl[][])
                n185 = local read "Display"() -> (w440:T7)
                n186 = Variant To Data(error in=w448, type=T15 {"Display"=enum."HOLOGRAM", "Plane number"=0} ("output cluster"), Variant=w447) -> (data=w445:T15, error out=w443:errorcluster)
                n187 = Unbundle(w445) -> ("Display"=w442:T7, "Plane number"=w444:u16)
                n188 = Select(t=w440, s=w443, f=w442) -> (s? t:f=w441:T7)
                n189 = case shown="\"HOLOGRAM\", Default" w441 {
                  tunnel: w453 -> [w474 w481 w501 w520 w540 w560 w580 w600]
                  tunnel: [w473 w497 w517 w537 w557 w577 w597 w617] -> w452
                  tunnel: w450 -> [w472 w496 w516 w536 w556 w576 w596 w616]
                  tunnel: w449 -> [w459 w485 w505 w525 w545 w565 w585 w605]
                  tunnel: w444 -> [_ w475 _ _ _ _ _ _]
                  frame "HOLOGRAM", Default {
                    n190 = call "HoloPy_get_hologram.vi"("Refnum in"=w474) -> ("error out"=w467:errorcluster, "HOLO_array"=w463:sgl[][])  [unwired: 8 in, 1 out]
                    n191 = local read "propagation"() -> (w471:T5)
                    n192 = local read "HoloParam"() -> (w468:T6)
                    n193 = Unbundle By Name(w468) -> ("pixel size"=w470:sgl, "objective magnification"=w469:sgl)
                    n194 = Unbundle By Name(w471) -> ("step"=w458:dbl)
                    n195 = Divide(x=w470, y=w469) -> (x/y=w457:sgl)
                    n196 = call "scaleFeaturesPositions_um_pix.vi"("error in (no error)"=w467, "dXY"=w457, "dZ"=w458, "FEATURES(µm)"=w459) -> ("error out"=w466:errorcluster, "Features(pix)"=w462:sgl[][])  [unwired: 6 in]
                    n197 = Bundle(cluster=T16 {"HOLO_array"=[], "FEATURES(µm)"=[], "Features(pix)"=[], "planeToDisplayFeatures"=enum."XY", "label"=""} ("output cluster"), "HOLO_array"=w463, "FEATURES(µm)"=w459, "Features(pix)"=w462, "planeToDisplayFeatures"=enum16{"XY", "XZ", "YZ"}."XY", "label"="Hologram" ("command")) -> (w461:T16)
                    n198 = Bundle By Name(cluster=cluster{"command":string, "data":variant} {"command"="updateDisplay", "data"=variant} ("element"), "data"=w461) -> (w464:cluster{"command":string, "data":variant})
                    n199 = Enqueue Element(queue=w472, element=w464, error in (no error)=w466) -> (error out=w473:errorcluster)  [unwired: 1 in, 2 out]
                  }
                  frame "XY PLANE NUMBER...." {
                    n200 = call "HoloPy_get_reconstruction_plane.vi"("plane number"=w475, "Refnum in"=w481) -> ("error out"=w480:errorcluster, "HOLO_array"=w479:sgl[][])  [unwired: 7 in, 1 out]
                    n201 = local read "propagation"() -> (w495:T5)
                    n202 = local read "HoloParam"() -> (w492:T6)
                    n203 = Unbundle By Name(w492) -> ("pixel size"=w494:sgl, "objective magnification"=w493:sgl)
                    n204 = Number To Decimal String(number=w475) -> (decimal integer string=w478:string)  [unwired: 1 in]
                    n205 = Unbundle By Name(w495) -> ("step"=w484:dbl)
                    n206 = Concatenate Strings("Hologram plane number " ("Label.Text"), w478) -> (w476:string)
                    n207 = Divide(x=w494, y=w493) -> (x/y=w483:sgl)
                    n208 = call "scaleFeaturesPositions_um_pix.vi"("error in (no error)"=w480, "dXY"=w483, "dZ"=w484, "FEATURES(µm)"=w485) -> ("error out"=w491:errorcluster, "Features(pix)"=w488:sgl[][])  [unwired: 6 in]
                    n209 = Bundle(cluster=T16 {"HOLO_array"=[], "FEATURES(µm)"=[], "Features(pix)"=[], "planeToDisplayFeatures"=enum."XY", "label"=""} ("output cluster"), "HOLO_array"=w479, "FEATURES(µm)"=w485, "Features(pix)"=w488, "planeToDisplayFeatures"=enum16{"XY", "XZ", "YZ"}."XY", "label"=w476) -> (w487:T16)
                    n210 = Bundle By Name(cluster=cluster{"command":string, "data":variant} {"command"="updateDisplay", "data"=variant} ("element"), "data"=w487) -> (w489:cluster{"command":string, "data":variant})
                    n211 = Enqueue Element(queue=w496, element=w489, error in (no error)=w491) -> (error out=w497:errorcluster)  [unwired: 1 in, 2 out]
                  }
                  frame "XY MAX PLANE" {
                    n212 = call "HoloPy_max_XY_planes_from_volume.vi"("Refnum in"=w501) -> ("error out"=w499:errorcluster, "XY Plane"=w500:sgl[][])  [unwired: 8 in, 1 out]
                    n213 = local read "propagation"() -> (w515:T5)
                    n214 = local read "HoloParam"() -> (w512:T6)
                    n215 = Unbundle By Name(w512) -> ("pixel size"=w514:sgl, "objective magnification"=w513:sgl)
                    n216 = Unbundle By Name(w515) -> ("step"=w504:dbl)
                    n217 = Divide(x=w514, y=w513) -> (x/y=w503:sgl)
                    n218 = call "scaleFeaturesPositions_um_pix.vi"("error in (no error)"=w499, "dXY"=w503, "dZ"=w504, "FEATURES(µm)"=w505) -> ("error out"=w511:errorcluster, "Features(pix)"=w508:sgl[][])  [unwired: 6 in]
                    n219 = Bundle(cluster=T16 {"HOLO_array"=[], "FEATURES(µm)"=[], "Features(pix)"=[], "planeToDisplayFeatures"=enum."XY", "label"=""} ("output cluster"), "HOLO_array"=w500, "FEATURES(µm)"=w505, "Features(pix)"=w508, "planeToDisplayFeatures"=enum16{"XY", "XZ", "YZ"}."XY", "label"="XY max focus plane projection" ("Label.Text")) -> (w507:T16)
                    n220 = Bundle By Name(cluster=cluster{"command":string, "data":variant} {"command"="updateDisplay", "data"=variant} ("element"), "data"=w507) -> (w509:cluster{"command":string, "data":variant})
                    n221 = Enqueue Element(queue=w516, element=w509, error in (no error)=w511) -> (error out=w517:errorcluster)  [unwired: 1 in, 2 out]
                  }
                  frame "XY SUM PLANE" {
                    n222 = call "HoloPy_sum_XY_planes_from_volume.vi"("Refnum in"=w520) -> ("error out"=w518:errorcluster, "XY Plane"=w519:sgl[][])  [unwired: 8 in, 1 out]
                    n223 = local read "propagation"() -> (w535:T5)
                    n224 = local read "HoloParam"() -> (w532:T6)
                    n225 = Unbundle By Name(w532) -> ("pixel size"=w534:sgl, "objective magnification"=w533:sgl)
                    n226 = Unbundle By Name(w535) -> ("step"=w524:dbl)
                    n227 = Divide(x=w534, y=w533) -> (x/y=w523:sgl)
                    n228 = call "scaleFeaturesPositions_um_pix.vi"("error in (no error)"=w518, "dXY"=w523, "dZ"=w524, "FEATURES(µm)"=w525) -> ("error out"=w531:errorcluster, "Features(pix)"=w528:sgl[][])  [unwired: 6 in]
                    n229 = Bundle(cluster=T16 {"HOLO_array"=[], "FEATURES(µm)"=[], "Features(pix)"=[], "planeToDisplayFeatures"=enum."XY", "label"=""} ("output cluster"), "HOLO_array"=w519, "FEATURES(µm)"=w525, "Features(pix)"=w528, "planeToDisplayFeatures"=enum16{"XY", "XZ", "YZ"}."XY", "label"="XY sum focus plane projection" ("Label.Text")) -> (w527:T16)
                    n230 = Bundle By Name(cluster=cluster{"command":string, "data":variant} {"command"="updateDisplay", "data"=variant} ("element"), "data"=w527) -> (w529:cluster{"command":string, "data":variant})
                    n231 = Enqueue Element(queue=w536, element=w529, error in (no error)=w531) -> (error out=w537:errorcluster)  [unwired: 1 in, 2 out]
                  }
                  frame "XZ MAX PLANE" {
                    n232 = call "HoloPy_max_XZ_planes_from_volume.vi"("Refnum in"=w540) -> ("error out"=w538:errorcluster, "XZ Plane"=w539:sgl[][])  [unwired: 8 in, 1 out]
                    n233 = local read "propagation"() -> (w555:T5)
                    n234 = local read "HoloParam"() -> (w552:T6)
                    n235 = Unbundle By Name(w552) -> ("pixel size"=w554:sgl, "objective magnification"=w553:sgl)
                    n236 = Unbundle By Name(w555) -> ("step"=w544:dbl)
                    n237 = Divide(x=w554, y=w553) -> (x/y=w543:sgl)
                    n238 = call "scaleFeaturesPositions_um_pix.vi"("error in (no error)"=w538, "dXY"=w543, "dZ"=w544, "FEATURES(µm)"=w545) -> ("error out"=w551:errorcluster, "Features(pix)"=w548:sgl[][])  [unwired: 6 in]
                    n239 = Bundle(cluster=T16 {"HOLO_array"=[], "FEATURES(µm)"=[], "Features(pix)"=[], "planeToDisplayFeatures"=enum."XY", "label"=""} ("output cluster"), "HOLO_array"=w539, "FEATURES(µm)"=w545, "Features(pix)"=w548, "planeToDisplayFeatures"=enum16{"XY", "XZ", "YZ"}."XZ", "label"="XZ  max focus plane projection" ("Label.Text")) -> (w547:T16)
                    n240 = Bundle By Name(cluster=cluster{"command":string, "data":variant} {"command"="updateDisplay", "data"=variant} ("element"), "data"=w547) -> (w549:cluster{"command":string, "data":variant})
                    n241 = Enqueue Element(queue=w556, element=w549, error in (no error)=w551) -> (error out=w557:errorcluster)  [unwired: 1 in, 2 out]
                  }
                  frame "XZ SUM PLANE" {
                    n242 = call "HoloPy_sum_XZ_planes_from_volume.vi"("Refnum in"=w560) -> ("error out"=w558:errorcluster, "XZ Plane"=w559:sgl[][])  [unwired: 8 in, 1 out]
                    n243 = local read "propagation"() -> (w575:T5)
                    n244 = local read "HoloParam"() -> (w572:T6)
                    n245 = Unbundle By Name(w572) -> ("pixel size"=w574:sgl, "objective magnification"=w573:sgl)
                    n246 = Unbundle By Name(w575) -> ("step"=w564:dbl)
                    n247 = Divide(x=w574, y=w573) -> (x/y=w563:sgl)
                    n248 = call "scaleFeaturesPositions_um_pix.vi"("error in (no error)"=w558, "dXY"=w563, "dZ"=w564, "FEATURES(µm)"=w565) -> ("error out"=w571:errorcluster, "Features(pix)"=w568:sgl[][])  [unwired: 6 in]
                    n249 = Bundle(cluster=T16 {"HOLO_array"=[], "FEATURES(µm)"=[], "Features(pix)"=[], "planeToDisplayFeatures"=enum."XY", "label"=""} ("output cluster"), "HOLO_array"=w559, "FEATURES(µm)"=w565, "Features(pix)"=w568, "planeToDisplayFeatures"=enum16{"XY", "XZ", "YZ"}."XZ", "label"="XZ  sum focus plane projection" ("Label.Text")) -> (w567:T16)
                    n250 = Bundle By Name(cluster=cluster{"command":string, "data":variant} {"command"="updateDisplay", "data"=variant} ("element"), "data"=w567) -> (w569:cluster{"command":string, "data":variant})
                    n251 = Enqueue Element(queue=w576, element=w569, error in (no error)=w571) -> (error out=w577:errorcluster)  [unwired: 1 in, 2 out]
                  }
                  frame "YZ MAX PLANE" {
                    n252 = call "HoloPy_max_YZ_planes_from_volume.vi"("Refnum in"=w580) -> ("error out"=w578:errorcluster, "YZ Plane"=w579:sgl[][])  [unwired: 8 in, 1 out]
                    n253 = local read "propagation"() -> (w595:T5)
                    n254 = local read "HoloParam"() -> (w592:T6)
                    n255 = Unbundle By Name(w592) -> ("pixel size"=w594:sgl, "objective magnification"=w593:sgl)
                    n256 = Unbundle By Name(w595) -> ("step"=w584:dbl)
                    n257 = Divide(x=w594, y=w593) -> (x/y=w583:sgl)
                    n258 = call "scaleFeaturesPositions_um_pix.vi"("error in (no error)"=w578, "dXY"=w583, "dZ"=w584, "FEATURES(µm)"=w585) -> ("error out"=w591:errorcluster, "Features(pix)"=w588:sgl[][])  [unwired: 6 in]
                    n259 = Bundle(cluster=T16 {"HOLO_array"=[], "FEATURES(µm)"=[], "Features(pix)"=[], "planeToDisplayFeatures"=enum."XY", "label"=""} ("output cluster"), "HOLO_array"=w579, "FEATURES(µm)"=w585, "Features(pix)"=w588, "planeToDisplayFeatures"=enum16{"XY", "XZ", "YZ"}."YZ", "label"="YZ max focus plane projection" ("Label.Text")) -> (w587:T16)
                    n260 = Bundle By Name(cluster=cluster{"command":string, "data":variant} {"command"="updateDisplay", "data"=variant} ("element"), "data"=w587) -> (w589:cluster{"command":string, "data":variant})
                    n261 = Enqueue Element(queue=w596, element=w589, error in (no error)=w591) -> (error out=w597:errorcluster)  [unwired: 1 in, 2 out]
                  }
                  frame "YZ SUM PLANE" {
                    n262 = call "HoloPy_sum_YZ_planes_from_volume.vi"("Refnum in"=w600) -> ("error out"=w598:errorcluster, "YZ Plane"=w599:sgl[][])  [unwired: 8 in, 1 out]
                    n263 = local read "propagation"() -> (w615:T5)
                    n264 = local read "HoloParam"() -> (w612:T6)
                    n265 = Unbundle By Name(w612) -> ("pixel size"=w614:sgl, "objective magnification"=w613:sgl)
                    n266 = Unbundle By Name(w615) -> ("step"=w604:dbl)
                    n267 = Divide(x=w614, y=w613) -> (x/y=w603:sgl)
                    n268 = call "scaleFeaturesPositions_um_pix.vi"("error in (no error)"=w598, "dXY"=w603, "dZ"=w604, "FEATURES(µm)"=w605) -> ("error out"=w611:errorcluster, "Features(pix)"=w608:sgl[][])  [unwired: 6 in]
                    n269 = Bundle(cluster=T16 {"HOLO_array"=[], "FEATURES(µm)"=[], "Features(pix)"=[], "planeToDisplayFeatures"=enum."XY", "label"=""} ("output cluster"), "HOLO_array"=w599, "FEATURES(µm)"=w605, "Features(pix)"=w608, "planeToDisplayFeatures"=enum16{"XY", "XZ", "YZ"}."YZ", "label"="YZ sum focus plane projection" ("Label.Text")) -> (w607:T16)
                    n270 = Bundle By Name(cluster=cluster{"command":string, "data":variant} {"command"="updateDisplay", "data"=variant} ("element"), "data"=w607) -> (w609:cluster{"command":string, "data":variant})
                    n271 = Enqueue Element(queue=w616, element=w609, error in (no error)=w611) -> (error out=w617:errorcluster)  [unwired: 1 in, 2 out]
                  }
                }
              }
              frame "displayHolo" {
                n272 = Unbundle By Name(w625) -> ("PythonSession"=w619:refnum<k35>)
                n273 = call "HoloPy_get_hologram.vi"("error in (no error)"=w621, "Refnum in"=w619) -> ("error out"=w620:errorcluster)  [unwired: 7 in, 2 out]
                n274 = Bundle By Name(cluster=w625, "LabelPicture"="Hologram" ("Label.Text"), "planeToDisplayFeatures"=enum16{"XY", "XZ", "YZ"}."XY", "Display"=TRUE) -> (w624:T12)
              }
              frame "displaySubVolume" {
                n275 = Unbundle By Name(w639) -> ("PythonSession"=w634:refnum<k35>)
                n276 = Variant To Data(error in=w633, type=T17 {"X"=0, "Y"=0, "Z"=0, "XYsize"=0, "ZSize"=0} ("param"), Variant=w632) -> (data=w630:T17, error out=w629:errorcluster)
                n277 = call "HoloPy_subvolume_3planes.vi"("error in (no error)"=w629, "param"=w630, "Refnum in"=w634) -> ("error out"=w635:errorcluster)  [unwired: 6 in, 2 out]
                n278 = Bundle By Name(cluster=w639, "LabelPicture"="sub volume 3 planes" ("Label.Text"), "planeToDisplayFeatures"=enum16{"XY", "XZ", "YZ"}."XY", "Display"=TRUE) -> (w638:T12)
              }
              frame "displayHolo_plane" {
                w646 = u16 0 ("Plane number")
                (unwired) "Hologram plane" ("Label.Text")
                n279 = Variant To Data(error in=w656, type=w646, Variant=w655) -> (data=w652:u16, error out=w654:errorcluster)
                n280 = Unbundle By Name(w651) -> ("PythonSession"=w653:refnum<k35>)
                n281 = call "HoloPy_get_reconstruction_plane.vi"("error in (no error)"=w654, "plane number"=w652, "Refnum in"=w653) -> ("error out"=w644:errorcluster)  [unwired: 6 in, 2 out]
                n282 = Number To Decimal String(number=w646) -> (decimal integer string=w645:string)  [unwired: 1 in]
                n283 = Concatenate Strings("Hologram plane number " ("Label.Text"), w645) -> (w647:string)
                n284 = Bundle By Name(cluster=w651, "LabelPicture"=w647, "planeToDisplayFeatures"=enum16{"XY", "XZ", "YZ"}."XY", "Display"=TRUE) -> (w650:T12)
              }
              frame "displayBin_plane" {
                w665 = u16 0 ("Plane number")
                n285 = Variant To Data(error in=w672, type=w665, Variant=w671) -> (data=w662:u16, error out=w663:errorcluster)
                n286 = Unbundle By Name(w670) -> ("PythonSession"=w661:refnum<k35>)
                n287 = call "HoloPy_get_binarised_plane.vi"("error in (no error)"=w663, "plane number"=w662, "Refnum in"=w661) -> ("error out"=w660:errorcluster)  [unwired: 6 in, 2 out]
                n288 = Number To Decimal String(number=w665) -> (decimal integer string=w664:string)  [unwired: 1 in]
                n289 = Concatenate Strings("Hologram bin plane number " ("Label.Text"), w664) -> (w666:string)
                n290 = Bundle By Name(cluster=w670, "LabelPicture"=w666, "planeToDisplayFeatures"=enum16{"XY", "XZ", "YZ"}."XY", "Display"=TRUE) -> (w669:T12)
              }
              frame "TEST SUM BIN PLANE" {
                n291 = Unbundle By Name(w682) -> ("PythonSession"=w677:refnum<k35>)
                n292 = call "HoloPy_get_sum_bin_planes.vi"("error in (no error)"=w676, "Refnum in"=w677) -> ("error out"=w679:errorcluster, "XY Plane"=w678:i32[][])  [unwired: 7 in, 1 out]
                n293 = To Single Precision Float(number=w678) -> ()  [unwired: 1 out]
                n294 = Bundle By Name(cluster=w682, "LabelPicture"="Sum thresholded planes" ("Label.Text"), "Display"=TRUE) -> (w681:T12)
              }
              frame "savePosition" {
                n295 = Variant To Data(error in=w693, type=path "" ("Holograms directory"), Variant=w692) -> (data=w687:path, error out=w690:errorcluster)
                n296 = Unbundle By Name(w686) -> ("PythonSession"=w688:refnum<k35>, "FEATURES(µm)"=w685:sgl[][])
                n297 = call "HoloPy_save_Features_csv.vi"("error in (no error)"=w690, "path csv file"=w687, "Array"=w685, "Refnum in"=w688) -> ("error out"=w689:errorcluster)  [unwired: 6 in, 1 out]
              }
            }
            n298 = Unbundle By Name(w93) -> ("State"=w92:T11)
            n299 = call "displayMessageSender.vi"("QueueTraitement"=w91, "error in (no error)"=w95, "DatasIN"=w93, "QueueMsgIN"=w97) -> ("error out"=w96:errorcluster, "DatasOUT"=w94:T12)  [unwired: 5 in, 1 out]
            n300 = global write "globState.vi" "State"(w92) -> ()
          }
          frame Error {
            n301 = flat-sequence {
              tunnel: w700 -> [w702]
              tunnel: w699 -> [w703]
              tunnel: [w703] -> w698
              tunnel: w698 -> [w705]
              frame #0 {
                n302 = Flush Queue(queue=w702) -> (queue out=w701:refnum<queue>)  [unwired: 1 in, 2 out]
                n303 = Enqueue Element(queue=w701, element=cluster{"command":string, "data":variant} {"command"="closePythonSession", "data"=variant}) -> ()  [unwired: 2 in, 3 out]
              }
              frame #1 {
                n304 = call <vilib>:"Simple Error Handler.vi"("error in (no error)"=w705) -> ()  [unwired: 4 in, 5 out]
              }
            }
          }
        }
      }
      n305 = while {
        tunnel: w82 -> [w709]
        tunnel: w81 -> [w708]
        tunnel: [w707] -> w80
        tunnel: w77 -> [w706]
        stop <- w710 stop-if-true
        # "USER EVENT"
        n306 = event shown="[5] \"Remove mean Hologram\", \"remove action\": Value Change" {
          selector: w708 -> [_ _ _ _ _ _ _ _ _ _ _ _ _ _]
          dyn-events: _ -> [_ _ _ _ _ _ _ _ _ _ _ _ _ _]
          timeout: _ -> [_ _ _ _ _ _ _ _ _ _ _ _ _ _]
          tunnel: [FALSE FALSE TRUE _ _ _ _ _ _ _ _ _ _ _] -> w710
          tunnel: w709 -> [w715 w723 _ w735 w762 w779 w791 w806 w816 w823 w831 w840 w842 w850]
          tunnel: [w711 w722 _ _ _ _ _ _ _ _ _ _ _ _] -> w707
          tunnel: w706 -> [w713 w717 _ _ _ _ _ _ _ _ _ _ _ _]
          event "EXIT": Value Change {
            w714 = cluster{"command":string, "data":variant} {"command"="EXIT", "data"=variant} ("element")
            n307 = event-data() -> ()  [unwired: 1 in, 1 out]
            n308 = Enqueue Element(queue=w715, element=w714) -> (error out=w712:errorcluster)  [unwired: 2 in, 2 out]
            n309 = Enqueue Element(queue=w713, element=w714, error in (no error)=w712) -> (error out=w711:errorcluster)  [unwired: 1 in, 2 out]
          }
          event Panel Close? {
            n310 = event-data() -> ()  [unwired: 1 in, 4 out]
            n311 = Two Button Dialog(message="EXIT APPLICATION?", 2:"YES" ("T button name (\"OK\")")) -> (T button?=w719:bool)  [unwired: 1 in]
            n312 = case shown="True" w719 {
              tunnel: w723 -> [_ w730]
              tunnel: [errorcluster {"status"=FALSE, "code"=0, "source"=""} ("error out") w726] -> w722
              tunnel: w717 -> [_ w728]
              frame False {
              }
              frame True {
                w727 = cluster{"command":string, "data":variant} {"command"="EXIT", "data"=variant} ("element")
                n313 = Enqueue Element(queue=w730, element=w727) -> (error out=w729:errorcluster)  [unwired: 2 in, 2 out]
                n314 = Enqueue Element(queue=w728, element=w727, error in (no error)=w729) -> (error out=w726:errorcluster)  [unwired: 1 in, 2 out]
              }
            }
            n315 = event-data("Discard?"=TRUE) -> ()  [unwired: 1 in, 1 out]
          }
          event User Event {
            n316 = event-data() -> ()  [unwired: 1 in, 5 out]
          }
          event "propagation": Value Change {
            n317 = event-data() -> ("OldVal"=w733:T5, "NewVal"=w732:T5)  [unwired: 1 in]
            n318 = global read "globState.vi" "State"() -> (w734:T11)
            n319 = case shown="\"TEST WAIT\"" w734 {
              tunnel: w735 -> [_ w741]
              tunnel: w733 -> [_ w740]
              tunnel: w732 -> [_ w739]
              frame "TEST IN PROGESS", Default {
              }
              frame "TEST WAIT" {
                n320 = Unbundle By Name(w740) -> ("number of planes"=w737:i32)
                n321 = Unbundle By Name(w739) -> ("number of planes"=w738:i32)
                n322 = Not Equal?(x=w737, y=w738) -> (x != y?=w736:bool)
                n323 = case shown="True" w736 {
                  tunnel: w741 -> [w744 w754]
                  frame False {
                    n324 = local read "Remove mean Hologram"() -> (w745:bool)
                    n325 = Select(t=string[] ["openHolo", "removeMeanHolo", "Display", "reconstructAndFocus", "computeThreshold", "findFeatures", "test finished", "Display"], s=w745, f=string[] ["openHolo", "Display", "reconstructAndFocus", "computeThreshold", "findFeatures", "test finished", "Display"]) -> (s? t:f=w746:string[])
                    n326 = for {
                      tunnel: w744 -> [w751]
                      tunnel: w746 -> [w749] mode=indexing
                      tunnel: [w747] -> _ mode=indexing
                      n327 = Bundle By Name(cluster=cluster{"command":string, "data":variant} {"command"="", "data"=variant} ("element"), "command"=w749) -> (w748:cluster{"command":string, "data":variant})
                      n328 = Enqueue Element(queue=w751, element=w748) -> (error out=w747:errorcluster)  [unwired: 2 in, 2 out]
                    }
                  }
                  frame True {
                    n329 = local read "Remove mean Hologram"() -> (w755:bool)
                    n330 = Select(t=string[] ["openPythonSession", "startTest", "allocate", "openHolo", "removeMeanHolo", "Display", "reconstructAndFocus", "computeThreshold", "findFeatures", "test finished", "Display"], s=w755, f=string[] ["openPythonSession", "startTest", "allocate", "openHolo", "Display", "reconstructAndFocus", "computeThreshold", "findFeatures", "test finished", "Display"]) -> (s? t:f=w756:string[])
                    n331 = for {
                      tunnel: w754 -> [w761]
                      tunnel: w756 -> [w759] mode=indexing
                      tunnel: [w757] -> _ mode=indexing
                      n332 = Bundle By Name(cluster=cluster{"command":string, "data":variant} {"command"="", "data"=variant} ("element"), "command"=w759) -> (w758:cluster{"command":string, "data":variant})
                      n333 = Enqueue Element(queue=w761, element=w758) -> (error out=w757:errorcluster)  [unwired: 2 in, 2 out]
                    }
                  }
                }
              }
            }
          }
          event "HoloDir": Value Change {
            n334 = event-data() -> ()  [unwired: 1 in, 6 out]
            n335 = global read "globState.vi" "State"() -> (w763:T11)
            n336 = case shown="\"TEST WAIT\"" w763 {
              tunnel: w762 -> [w764 w767]
              frame "WAIT", Default {
                n337 = Enqueue Element(queue=w764, element=cluster{"command":string, "data":variant} {"command"="clear mean holo", "data"=variant}) -> ()  [unwired: 2 in, 3 out]
              }
              frame "TEST WAIT" {
                n338 = Enqueue Element(queue=w767, element=cluster{"command":string, "data":variant} {"command"="clear mean holo", "data"=variant}) -> (queue out=w766:refnum<queue>)  [unwired: 2 in, 2 out]
                n339 = local read "Remove mean Hologram"() -> (w771:bool)
                n340 = Select(t=string[] ["openPythonSession", "startTest", "allocate", "get holo path list", "openHolo", "Display", "get holo path list", "computeMeanHolo", "removeMeanHolo", "Display", "reconstructAndFocus", "computeThreshold", "findFeatures", "test finished", "Display"], s=w771, f=string[] ["openPythonSession", "startTest", "allocate", "get holo path list", "openHolo", "Display", "reconstructAndFocus", "computeThreshold", "findFeatures", "test finished", "Display"]) -> (s? t:f=w772:string[])
                n341 = for {
                  tunnel: w766 -> [w777]
                  tunnel: w772 -> [w775] mode=indexing
                  tunnel: [w773] -> _ mode=indexing
                  n342 = Bundle By Name(cluster=cluster{"command":string, "data":variant} {"command"="", "data"=variant} ("element"), "command"=w775) -> (w774:cluster{"command":string, "data":variant})
                  n343 = Enqueue Element(queue=w777, element=w774) -> (error out=w773:errorcluster)  [unwired: 2 in, 2 out]
                }
              }
            }
          }
          event "Remove mean Hologram", "remove action": Value Change {
            n344 = event-data() -> ()  [unwired: 1 in, 6 out]
            n345 = global read "globState.vi" "State"() -> (w778:T11)
            n346 = case shown="\"TEST WAIT\"" w778 {
              tunnel: w779 -> [_ w782]
              frame "TEST IN PROGESS", Default {
              }
              frame "TEST WAIT" {
                n347 = local read "Remove mean Hologram"() -> (w783:bool)
                n348 = Select(t=string[] ["openHolo", "computeMeanHolo", "removeMeanHolo", "Display", "reconstructAndFocus", "computeThreshold", "findFeatures", "test finished", "Display"], s=w783, f=string[] ["openHolo", "Display", "reconstructAndFocus", "computeThreshold", "findFeatures", "test finished", "Display"]) -> (s? t:f=w784:string[])
                n349 = for {
                  tunnel: w782 -> [w789]
                  tunnel: w784 -> [w787] mode=indexing
                  tunnel: [w785] -> _ mode=indexing
                  n350 = Bundle By Name(cluster=cluster{"command":string, "data":variant} {"command"="", "data"=variant} ("element"), "command"=w787) -> (w786:cluster{"command":string, "data":variant})
                  n351 = Enqueue Element(queue=w789, element=w786) -> (error out=w785:errorcluster)  [unwired: 2 in, 2 out]
                }
              }
            }
          }
          event "hologram to test": Value Change {
            n352 = event-data() -> ()  [unwired: 1 in, 6 out]
            n353 = global read "globState.vi" "State"() -> (w790:T11)
            n354 = case shown="\"TEST WAIT\"" w790 {
              tunnel: w791 -> [_ w794]
              frame "TEST IN PROGESS", Default {
              }
              frame "TEST WAIT" {
                n355 = local read "Remove mean Hologram"() -> (w795:bool)
                n356 = Select(t=string[] ["change holo", "openHolo", "removeMeanHolo", "Display", "reconstructAndFocus", "computeThreshold", "findFeatures", "test finished", "Display"], s=w795, f=string[] ["change holo", "openHolo", "Display", "reconstructAndFocus", "computeThreshold", "findFeatures", "test finished", "Display"]) -> (s? t:f=w796:string[])
                n357 = for {
                  tunnel: w794 -> [w801]
                  tunnel: w796 -> [w799] mode=indexing
                  tunnel: [w797] -> _ mode=indexing
                  n358 = Bundle By Name(cluster=cluster{"command":string, "data":variant} {"command"="", "data"=variant} ("element"), "command"=w799) -> (w798:cluster{"command":string, "data":variant})
                  n359 = Enqueue Element(queue=w801, element=w798) -> (error out=w797:errorcluster)  [unwired: 2 in, 2 out]
                }
              }
            }
          }
          event "testMode": Value Change {
            n360 = event-data() -> ()  [unwired: 1 in, 6 out]
            n361 = Select(t=string[] ["openPythonSession", "startTest", "allocate", "get holo path list", "openHolo", "Display", "computeMeanHolo", "removeMeanHolo", "Display", "reconstructAndFocus", "computeThreshold", "findFeatures", "test finished", "Display"] ("old"), s="Remove mean Hologram", f=string[] ["openPythonSession", "startTest", "allocate", "get holo path list", "openHolo", "Display", "reconstructAndFocus", "computeThreshold", "findFeatures", "test finished", "Display"]) -> (s? t:f=w805:string[])
            n362 = for {
              tunnel: w806 -> [w811]
              tunnel: w805 -> [w809] mode=indexing
              tunnel: [w807] -> _ mode=indexing
              n363 = Bundle By Name(cluster=cluster{"command":string, "data":variant} {"command"="", "data"=variant} ("element"), "command"=w809) -> (w808:cluster{"command":string, "data":variant})
              n364 = Enqueue Element(queue=w811, element=w808) -> (error out=w807:errorcluster)  [unwired: 2 in, 2 out]
            }
          }
          event "BATCH": Value Change {
            n365 = event-data() -> ()  [unwired: 1 in, 6 out]
            n366 = local read "Remove mean Hologram"() -> (w814:bool)
            n367 = Select(t=string[] ["openPythonSession", "statusBatch", "allocate", "get holo path list", "computeMeanHolo", "start batch"], s=w814, f=string[] ["openPythonSession", "statusBatch", "allocate", "get holo path list", "start batch"]) -> (s? t:f=w815:string[])
            n368 = for {
              tunnel: w816 -> [w821]
              tunnel: w815 -> [w819] mode=indexing
              tunnel: [w817] -> _ mode=indexing
              n369 = Bundle By Name(cluster=cluster{"command":string, "data":variant} {"command"="", "data"=variant} ("element"), "command"=w819) -> (w818:cluster{"command":string, "data":variant})
              n370 = Enqueue Element(queue=w821, element=w818) -> (error out=w817:errorcluster)  [unwired: 2 in, 2 out]
            }
          }
          event "Fourier BP filter (pix)", "Focus": Value Change {
            n371 = event-data() -> ()  [unwired: 1 in, 1 out]
            n372 = global read "globState.vi" "State"() -> (w822:T11)
            n373 = case shown="\"WAIT\", Default" w822 {
              tunnel: w823 -> [_ w825]
              frame "WAIT", Default {
              }
              frame "TEST WAIT" {
                n374 = for {
                  tunnel: w825 -> [w830]
                  tunnel: string[] ["setParam", "reconstructAndFocus", "computeThreshold", "findFeatures", "test finished", "Display"] -> [w828] mode=indexing
                  tunnel: [w826] -> _ mode=indexing
                  n375 = Bundle By Name(cluster=cluster{"command":string, "data":variant} {"command"="", "data"=variant} ("element"), "command"=w828) -> (w827:cluster{"command":string, "data":variant})
                  n376 = Enqueue Element(queue=w830, element=w827) -> (error out=w826:errorcluster)  [unwired: 2 in, 2 out]
                }
              }
            }
          }
          event "exitTestMode": Value Change {
            n377 = event-data() -> ()  [unwired: 1 in, 6 out]
            n378 = Flush Queue(queue=w831) -> (queue out=w833:refnum<queue>)  [unwired: 1 in, 2 out]
            n379 = for {
              tunnel: w833 -> [w838]
              tunnel: string[] ["stopTest", "closePythonSession"] -> [w836] mode=indexing
              tunnel: [w834] -> _ mode=indexing
              n380 = Bundle By Name(cluster=cluster{"command":string, "data":variant} {"command"="", "data"=variant} ("element"), "command"=w836) -> (w835:cluster{"command":string, "data":variant})
              n381 = Enqueue Element(queue=w838, element=w835) -> (error out=w834:errorcluster)  [unwired: 2 in, 2 out]
            }
          }
          event "CANCEL_BATCH": Value Change {
            n382 = event-data() -> ()  [unwired: 1 in, 6 out]
            n383 = Enqueue Element At Opposite End(queue=w840, element=cluster{"command":string, "data":variant} {"command"="cancelBatch", "data"=variant}) -> ()  [unwired: 2 in, 3 out]
          }
          event "Display", "Plane number": Value Change {
            n384 = event-data() -> ()  [unwired: 1 in, 6 out]
            n385 = global read "globState.vi" "State"() -> (w841:T11)
            n386 = case shown="\"TEST WAIT\"" w841 {
              tunnel: w842 -> [_ _ w848 _ _]
              frame "SESSION CLOSED", Default {
              }
              frame "WAIT" {
              }
              frame "TEST WAIT" {
                n387 = Bundle("Display"="Display", "Plane number"="Plane number") -> (w845:T15)  [unwired: 1 in]
                n388 = Bundle By Name(cluster=cluster{"command":string, "data":variant} {"command"="Display", "data"=variant} ("element"), "data"=w845) -> (w844:cluster{"command":string, "data":variant})
                n389 = Enqueue Element(queue=w848, element=w844) -> ()  [unwired: 2 in, 3 out]
              }
              frame "TEST IN PROGESS" {
              }
              frame "BATCH IN PROGRESS" {
              }
            }
          }
          event Key Down {
            n390 = event-data() -> ("VKey"=w851:T18)  [unwired: 1 in, 8 out]
            n391 = local read "propagation"() -> (w849:T5)
            n392 = case shown="\"PageUp\"" w851 {
              tunnel: w850 -> [_ w852 w866]
              tunnel: w849 -> [_ _ w865]
              frame "ASCII", Default {
              }
              frame "PageDown" {
                n393 = global read "globState.vi" "State"() -> (w853:T11)
                n394 = case shown="\"TEST WAIT\"" w853 {
                  tunnel: w852 -> [_ _ w857 _ _]
                  frame "SESSION CLOSED", Default {
                  }
                  frame "WAIT" {
                  }
                  frame "TEST WAIT" {
                    n395 = local read "Plane number"() -> (w856:u16)
                    n396 = Decrement(x=w856) -> (x-1=w855:u16)
                    n397 = Greater Than 0?(x=w855) -> (x > 0?=w854:bool)
                    n398 = case shown="True" w854 {
                      tunnel: w857 -> [_ w863]
                      tunnel: w855 -> [_ w859]
                      frame False {
                      }
                      frame True {
                        n399 = local read "Display"() -> (w858:T7)
                        n400 = Bundle("Display"=w858, w859) -> (w862:T19)  [unwired: 1 in]
                        n401 = Bundle By Name(cluster=cluster{"command":string, "data":variant} {"command"="Display", "data"=variant} ("element"), "data"=w862) -> (w861:cluster{"command":string, "data":variant})
                        n402 = local write "Plane number"(w859) -> ()
                        n403 = Enqueue Element(queue=w863, element=w861) -> ()  [unwired: 2 in, 3 out]
                      }
                    }
                  }
                  frame "TEST IN PROGESS" {
                  }
                  frame "BATCH IN PROGRESS" {
                  }
                }
              }
              frame "PageUp" {
                n404 = Unbundle By Name(w865) -> ("number of planes"=w864:i32)
                n405 = global read "globState.vi" "State"() -> (w867:T11)
                n406 = case shown="\"TEST WAIT\"" w867 {
                  tunnel: w866 -> [_ _ w872 _ _]
                  tunnel: w864 -> [_ _ w868 _ _]
                  frame "SESSION CLOSED", Default {
                  }
                  frame "WAIT" {
                  }
                  frame "TEST WAIT" {
                    n407 = local read "Plane number"() -> (w871:u16)
                    n408 = Increment(x=w871) -> (x+1=w869:u16)
                    n409 = Less?(x=w869, y=w868) -> (x < y?=w870:bool)
                    n410 = case shown="True" w870 {
                      tunnel: w872 -> [_ w878]
                      tunnel: w869 -> [_ w874]
                      frame False {
                      }
                      frame True {
                        n411 = local read "Display"() -> (w873:T7)
                        n412 = Bundle("Display"=w873, w874) -> (w877:T19)  [unwired: 1 in]
                        n413 = Bundle By Name(cluster=cluster{"command":string, "data":variant} {"command"="Display", "data"=variant} ("element"), "data"=w877) -> (w876:cluster{"command":string, "data":variant})
                        n414 = local write "Plane number"(w874) -> ()
                        n415 = Enqueue Element(queue=w878, element=w876) -> ()  [unwired: 2 in, 3 out]
                      }
                    }
                  }
                  frame "TEST IN PROGESS" {
                  }
                  frame "BATCH IN PROGRESS" {
                  }
                }
              }
            }
          }
        }
      }
      n416 = while {
        tunnel: w77 -> [w887]
        tunnel: w79 -> [w881]
        tunnel: [w880] -> w76
        tunnel: w74 -> [w879]
        stop <- w882 stop-if-true
        # "DISPLAY AND SAVE"
        n417 = Dequeue Element(queue=w887) -> (element=w885:cluster{"command":string, "data":variant}, error out=w886:errorcluster)  [unwired: 2 in, 2 out]
        n418 = Unbundle(w885) -> ("command"=w884:string, "data"=w883:variant)
        n419 = case shown="\"updateDisplay\"" w884 {
          tunnel: w886 -> [w888 w895 w903 w919 w940 w941]
          tunnel: w883 -> [_ w894 w902 w918 w939 _]
          tunnel: [FALSE FALSE FALSE FALSE FALSE TRUE] -> w882
          tunnel: w881 -> [_ _ _ _ _ w943]
          tunnel: [w888 w891 w900 w914 w937 w941] -> w880
          tunnel: w879 -> [_ _ w898 _ _ _]
          frame "", Default {
          }
          frame "updateStatus" {
            n420 = Variant To Data(error in=w895, type="" ("return value"), Variant=w894) -> (data=→"Status":string, error out=w891:errorcluster)
          }
          frame "updateBtnIHM" {
            n421 = Variant To Data(error in=w903, type=T11."SESSION CLOSED" ("State"), Variant=w902) -> (data=w897:T11, error out=w899:errorcluster)
            n422 = call "activateBtnIHM.vi"("error in (no error)"=w899, "State"=w897, "References"=w898) -> ("error out"=w900:errorcluster)  [unwired: 8 in]
          }
          frame "updateDisplay" {
            n423 = Variant To Data(error in=w919, type=T16 {"HOLO_array"=[], "FEATURES(µm)"=[], "Features(pix)"=[], "planeToDisplayFeatures"=enum."XY", "label"=""} ("output cluster"), Variant=w918) -> (data=w916:T16, error out=w906:errorcluster)
            n424 = Unbundle(w916) -> ("HOLO_array"=w904:sgl[][], "FEATURES(µm)"=w910:sgl[][], "Features(pix)"=w905:sgl[][], "planeToDisplayFeatures"=w907:enum16{"XY", "XZ", "YZ"}, "label"=w908:string)
            n425 = Not Equal?(x=w910, y=sgl[][] []) -> (x != y?=w912:bool)
            n426 = case shown="True" w912 {
              tunnel: w910 -> [_ w923]
              frame False {
              }
              frame True {
                w927 = 1000000.0
                n427 = Array Subset(array=w923, index (col)=1 ("index"), length (col)=3 ("length")) -> (→"objects positions":sgl[][])  [unwired: 2 in]
                n428 = Index Array(array=w923, index (col) #1=1 ("disabled index (col)"), index (col) #2=2 ("index (col)"), index (col) #3=3 ("index (col)")) -> (element #1=w928:sgl[], element #2=w929:sgl[], element #3=w930:sgl[])  [unwired: 3 in]
                n429 = Multiply(x=w929, y=w927) -> (x*y=w933:dbl[])
                n430 = Multiply(x=w928, y=w927) -> (x*y=w932:dbl[])
                n431 = Multiply(x=w930, y=w927) -> (x*y=w931:dbl[])
                n432 = call-poly <vilib>:"Plot Helper.vi"("z vector"=w931, "y vector"=w932, "x vector"=w933) -> ("3D Plot lvclass Array out"=→"3D Scatter":refnum<class "3D Plot Datatype.lvclass">[])  [unwired: 3 in, 5 out]
              }
            }
            n433 = control-ref of="2D Picture"() -> (w915:refnum<vi>)
            n434 = call "convert_float_array_to_U8_Picture.vi"("Pict Refnum"=w915, "error in (no error)"=w906, "planeToDisplayFeatures"=w907, "FEATURES (PIX)"=w905, "HOLO"=w904) -> ("error out"=w914:errorcluster, "new picture"=→"2D Picture":picture)  [unwired: 5 in]
            n435 = property on="2D Picture" class="Pict"("Caption.Text"=w908) -> ()  [unwired: 2 in, 2 out]
          }
          frame "updateLabelPicture" {
            n436 = Variant To Data(error in=w940, type="label" ("Label.Text"), Variant=w939) -> (data=w935:string, error out=w937:errorcluster)
            n437 = property on="2D Picture" class="Pict"("Caption.Text"=w935) -> ()  [unwired: 2 in, 2 out]
          }
          frame "EXIT" {
            n438 = Generate User Event(user event=w943, event data cluster=TRUE ("event data")) -> ()  [unwired: 2 in, 2 out]
          }
        }
      }
    }
    frame #2 {
      n439 = local read "Batch threshold"() -> (w956:T3)
      n440 = local read "Fourier BP filter (pix)"() -> (w954:T1)
      n441 = local read "PythonVer"() -> (w948:string)
      n442 = local read "Python/Environnement\npath"() -> (w949:path)
      n443 = local read "HoloDir"() -> (w950:path)
      n444 = local read "HoloParam"() -> (w951:T6)
      n445 = local read "Remove mean Hologram"() -> (w952:bool)
      n446 = local read "propagation"() -> (w953:T5)
      n447 = local read "Focus"() -> (w955:T4)
      n448 = local read "CCL parameters"() -> (w957:T2)
      n449 = Merge Errors(w960, w961, w962) -> (w959:errorcluster)
      n450 = Destroy User Event(user event=w963, error in=w959) -> (error out=w965:errorcluster)
      n451 = Unregister For Events(event registration refnum=w964, error in=w965) -> (error out=w945:errorcluster)
      n452 = Bundle("PythonVer"=w948, "Python/Environnement\npath"=w949, "HoloDir"=w950, "HoloParam"=w951, "Remove mean Hologram"=w952, "propagation"=w953, "Fourier BP filter (pix)"=w954, "Focus"=w955, "Batch threshold"=w956, "CCL parameters"=w957) -> (w958:T20)  [unwired: 1 in]
      n453 = call "EcrireLireValeurParDefaut_HoloTrackPy_locate.vi"("Lecture/Ecriture"=enum32{"Lecture", "Ecriture"}."Ecriture", "ParamIN"=w958) -> ("error out"=w946:errorcluster)  [unwired: 6 in, 3 out]
      n454 = disable-structure shown="RUN_TIME_ENGINE==True" {
        disable-tunnel: w946 -> [_ _]
        disable-tunnel: w945 -> [_ _]
        frame condition #0 {
          n455 = Quit LabVIEW(quit? (T)=TRUE) -> ()
        }
        frame condition #1 (active) {
        }
      }
    }
  }
